vi "Process.vi"(8 "error in":errorcluster, 11 "LockinDAQ":refnum<class "Lockin.DAQ.lvclass">) -> (0 "error out":errorcluster, 3 "LockinDAQ out":refnum<class "Lockin.DAQ.lvclass">)   [LabVIEW 2016, in "Lockin.DAQ.lvclass"]
doc: "---------------------------------------------------------------\nJKI State Machine Objects™\nhttp://jki.net/state-machine-objects/\nCopyright (C) 2005-2015, JKI <info@jki.net>\nALL RIGHTS RESERVED"
uses:
  Lockin.DAQ.lvclass
  C:/Program Files (x86)/National Instruments/LabVIEW 2016/vi.lib/JKI/JKI SMO/SMO/SMO.lvclass
  Typedefs/State-enum.ctl
  <vilib>/JKI/JKI SMO/SMO/Typedefs/Parent Call--Enum.ctl
  Lockin.DAQ.lvclass/Lockin.DAQ.ctl
  Typedefs/Results--Cluster.ctl
  Typedefs/Sample Mode--Ring.ctl
  Typedefs/SweepResults--Cluster.ctl
  Typedefs/PublicEvents--Lockin.DAQ.getSweepWaveforms.ctl
  Typedefs/PrivateEvents--Cluster.ctl
  Typedefs/PrivateEvents--Lockin.DAQ.setAOconfig.ctl
  Typedefs/AO.config-array.ctl
  Typedefs/AO.config-cluster.ctl
  Typedefs/446xAO-enum.ctl
  Typedefs/DAQType-enum.ctl
  Typedefs/PrivateEvents--Lockin.DAQ.setAIconfig.ctl
  Typedefs/AI.config-array.ctl
  Typedefs/AI.config-cluster.ctl
  Typedefs/AI.coupling-enum.ctl
  Typedefs/446xAI-enum.ctl
  Typedefs/AI Simulation-enum.ctl
  Typedefs/PrivateEvents--Lockin.DAQ.setAO.ctl
  Typedefs/AO-cluster.ctl
  Instrument.Lockinl.UI/Typedefs/AO Channel--Cluster.ctl
  Typedefs/Function-enum.ctl
  Typedefs/PrivateEvents--Lockin.DAQ.setREF.ctl
  Typedefs/REF-cluster.ctl
  Instrument.Lockinl.UI/Typedefs/REF Channel--Cluster.ctl
  Typedefs/PrivateEvents--Lockin.DAQ.setSampling.ctl
  Typedefs/Sampling.ctl
  Typedefs/PrivateEvents--Lockin.DAQ.setState.ctl
  Typedefs/Set State-enum.ctl
  Typedefs/PrivateEvents--Lockin.DAQ.setInputGain.ctl
  Typedefs/PrivateEvents--Lockin.DAQ.setSweep.ctl
  Typedefs/Sweep Configuration--Cluster.ctl
  Instrument.Lockinl.UI/Typedefs/Sweep Channel--Cluster.ctl
  Typedefs/Sweep Pattern--Enum.ctl
  Typedefs/PrivateEvents--Lockin.DAQ.measureOffset.ctl
  Typedefs/PrivateEvents--Lockin.DAQ.zeroOffset.ctl
  Typedefs/PrivateEvents--Lockin.DAQ.setPreFilter.ctl
  Typedefs/AI Prefilter-cluster.ctl
  Typedefs/PrivateEvents--Lockin.DAQ.autoContigureDAQ.ctl
  Typedefs/PrivateEvents--LockinDAQ.setCalibration.ctl
  Typedefs/PrivateEvents--Lockin.DAQ.setAI.ctl
  Typedefs/AI-cluster.ctl
  Instrument.Lockinl.UI/Typedefs/AI Channel--Cluster.ctl
  Typedefs/PrivateEvents--Lockin.DAQ.Reset Phase.ctl
  <vilib>/JKI/JKI SMO/SMO/Typedefs/Protected Events.ctl
  <vilib>/JKI/JKI SMO/SMO/Typedefs/StopProcessEventData--Cluster.ctl
  <vilib>/JKI/JKI SMO/SMO/Typedefs/AbortProcessEventData--Cluster.ctl
  <vilib>/JKI/JKI SMO/SMO/Typedefs/SMO Dependency Event--Cluster.ctl
  <vilib>/JKI/JKI SMO/SMO/Typedefs/SMO Dependency Event--Enum.ctl
  <vilib>/Analysis/2dsp.llb/Decimate (single shot).vi
  <vilib>/Analysis/2dsp.llb/Decimate (single shot, DBL).vi
  <vilib>/Utility/High Resolution Relative Seconds.vi
  <vilib>/Waveform/WDTOps.llb/Number of Waveform Samples.vi
  <vilib>/Waveform/WDTOps.llb/WDT Number of Waveform Samples DBL.vi
  <vilib>/measure/madcrms.llb/Basic Averaged DC-RMS for N Chan.vi
  <vilib>/JKI/JKI SMO/SMO/SMO.lvclass
  <resource>/objmgr/daqmx.rc
  Instrument.Lockin/Instrument.Lockin.lvclass
  <vilib>/measure/NI_MAPro.lvlib
  Instrument.Lockinl.UI/Instrument.Lockin.UI.lvclass
panel:
  in  "Tab Control":enum32{"SMO", "Other", "Sweeping"}(tab)
  out "DAQ state":T1=enum."created"
  out "Method":string
  out "to":i32
  in  "LP Cutoff (Hz)":dbl=0.45 format="%#_13g"
  in  "LP filter?":bool
  in  "60 Hz Prefilter?":bool
  in  "reset REF":bool
  out "DAQ Create Tasks (ms)":u32
  out "DAQ AO/AI (ms)":u32
  out "Lockin (ms)":u32
  out "WFM Generation (ms)":u32
  out "DAQ Start Tasks (ms)":u32
  out "Payload":variant
  out "State":string
  in  "measure offset":bool
  in  "zero offset":bool
  in  "Reset Phase?":bool
  in  "autophase?\n(experimental)":bool
  out "ms":u32
  out "Sweeping Time":timestamp
  out "Sweep Start":timestamp
  out "Sweep Wait Time":timestamp
  out "sweeping":dbl
  out "sweep index":i32
  out "waiting (s)":dbl
  out "done sweep?":bool
  out "timeout?":bool
  # "For instructions on how to use the JKI State Machine Objects, examples and video tutorials, visit:\nhttp://jki.net/state-machine-objects/\n\nJKI State Machine Objects™\nhttp://jki.net/state-machine-objects/\nCopyright (C) 2005-2015, JKI <info@jki.net>\nALL RIGHTS RESERVED"
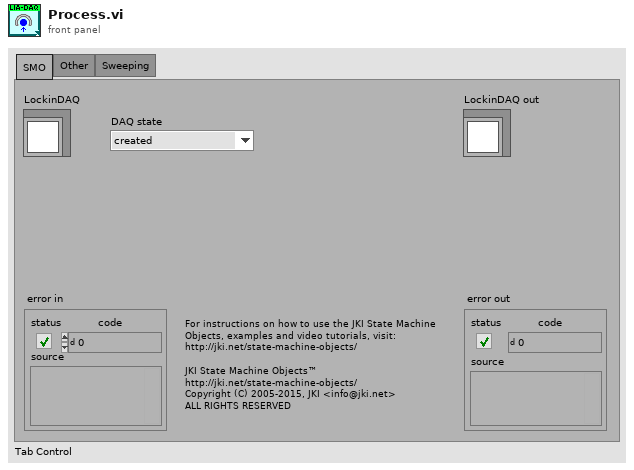
[diagram p1: front panel]
types:
  T1 = typedef "Lockin.DAQ.lvclass/State-enum.ctl" = enum16{"idle", "created", "started", "stopped", "sweeping"}
  T2 = typedef "SMO.lvclass/Parent Call--Enum.ctl" = enum16{"Allows parent to run", "Does not request parent to run"}
  T3 = enum32{"invalid app kind", "Development System", "Run Time System", "Student Edition", "Embedded LabVIEW", "Evaluation", "Custom"}
  T4 = enum32{"Invalid", "Standard", "Closed", "Hidden", "Minimized", "Maximized"}
  T5 = enum32{"Bad", "Idle", "Run top level", "Running"}
  T6 = typedef "Lockin.DAQ.lvclass/SweepResults--Cluster.ctl" = cluster{"X results":waveform(dbl)[], "Y Results":waveform(dbl)[]}
  T7 = typedef "Lockin.DAQ.lvclass/Sample Mode--Ring.ctl" = i32
  T8 = typedef "Lockin.DAQ.lvclass/AO.config-array.ctl" = T9[]
  T9 = typedef "Lockin.DAQ.lvclass/AO.config-cluster.ctl" = cluster{"AO.channels":tag, "AO.Range":T10, "output terminal configuration":i32, "DAQ Type":T11}
  T10 = typedef "Lockin.DAQ.lvclass/446xAO-enum.ctl" = enum16{"±0.1", "±1.0", "±10.0"}
  T11 = typedef "Lockin.DAQ.lvclass/DAQType-enum.ctl" = enum16{"None", "USB 4431", "PXI 446x"}
  T12 = typedef "Lockin.DAQ.lvclass/Results--Cluster.ctl" = cluster{"Time Stamp":timestamp, "Results":dbl[][]}
  T13 = cluster{"Core":cluster{"Current VI Reference":refnum<vi>, "Close Panel on Exit?":bool, "error":errorcluster}, "Self Reference":refnum<class "Lockin.DAQ.lvclass">, "to":i32, "state":T1, "sample mode":T7, "AO":waveform(dbl)[], "AI":waveform(dbl)[], "Reference":cluster{"X":waveform(dbl)[], "Y":waveform(dbl)[]}, "Results":T12, "sweep index":i32, "SweepResults [i]":T6, "SweepResults []":T6, "DAQ Offset":dbl[], "Sweep_AO":waveform(dbl)[], "Sweep_AI":waveform(dbl)[], "Reset Phase":bool, "Measure Offset":bool}
  T14 = typedef "Lockin.DAQ.lvclass/AI.config-array.ctl" = T15[]
  T15 = typedef "Lockin.DAQ.lvclass/AI.config-cluster.ctl" = cluster{"AI.channels":tag, "AI.Coupling":T16, "AI.Range":T17, "input terminal configuration":i32, "DAQ Type":T11}
  T16 = typedef "Lockin.DAQ.lvclass/AI.coupling-enum.ctl" = u16
  T17 = typedef "Lockin.DAQ.lvclass/446xAI-enum.ctl" = enum16{"±0.316", "±1.00", "±3.16", "±10.0", "±31.6", "±42.4"}
  T18 = typedef "Lockin.DAQ.lvclass/AI Simulation-enum.ctl" = enum16{"AI = HW simulated", "AI = noise*AO", "AI = waveguide"}
  T19 = cluster{"AI Configuration":T14, "Simulation mode":T18}
  T20 = typedef "Lockin.DAQ.lvclass/AO-cluster.ctl" = T21[]
  T21 = typedef "Instrument.Lockin.UI.lvclass/AO Channel--Cluster.ctl" = cluster{"Enable?":bool, "Channel":i32, "Amplitude":dbl, "Offset":dbl, "Frequency":dbl, "Phase":dbl, "Function":T22, "Sweeping?":bool}
  T22 = typedef "Lockin.DAQ.lvclass/Function-enum.ctl" = enum16{"Sine", "Triangle", "Square"}
  T23 = typedef "Lockin.DAQ.lvclass/AI-cluster.ctl" = T24[]
  T24 = typedef "Instrument.Lockin.UI.lvclass/AI Channel--Cluster.ctl" = cluster{"Enable?":bool, "Channel":i32, "References":u16[]}
  T25 = typedef "Lockin.DAQ.lvclass/REF-cluster.ctl" = T26[]
  T26 = typedef "Instrument.Lockin.UI.lvclass/REF Channel--Cluster.ctl" = cluster{"Enable?":bool, "Channel":i32, "Frequency":dbl, "Phase":dbl, "TC":dbl, "Order":i32}
  T27 = typedef "Lockin.DAQ.lvclass/PrivateEvents--Lockin.DAQ.setInputGain.ctl" = dbl[]
  T28 = typedef "Lockin.DAQ.lvclass/Sampling.ctl" = cluster{"Fs":dbl, "#s":i32}
  T29 = cluster{"Sampling":T28, "Sample Mode":T7, "AI Buffer Size (S)":i32, "Decimation":i32}
  T30 = typedef "Lockin.DAQ.lvclass/Sweep Configuration--Cluster.ctl" = cluster{"Sweep Time (s)":dbl, "Initial Wait (s)":dbl, "Return to Start":bool, "Channels":T31[]}
  T31 = typedef "Instrument.Lockin.UI.lvclass/Sweep Channel--Cluster.ctl" = cluster{"End":dbl, "Start":dbl, "Channel":u16, "Pattern":T32}
  T32 = typedef "Lockin.DAQ.lvclass/Sweep Pattern--Enum.ctl" = enum16{"Ramp /", "Ramp /\\", "Smooth Ramp _/", "Smooth Ramp _/\\_", "Frequency"}
  T33 = typedef "Lockin.DAQ.lvclass/PrivateEvents--Lockin.DAQ.measureOffset.ctl" = bool
  T34 = typedef "Lockin.DAQ.lvclass/PrivateEvents--Lockin.DAQ.Reset Phase.ctl" = bool
  T35 = typedef "Lockin.DAQ.lvclass/AI Prefilter-cluster.ctl" = cluster{"60 Hz prefilter":bool, "LP prefilter":bool, "LP cutoff (Hz)":dbl}
  T36 = typedef "Lockin.DAQ.lvclass/Set State-enum.ctl" = enum16{"start", "stop", "reset", "start sweep", "stop sweep"}
  T37 = typedef "Lockin.DAQ.lvclass/PrivateEvents--LockinDAQ.setCalibration.ctl" = bool
  T38 = cluster{"X":waveform(dbl)[], "Y":waveform(dbl)[]}
  T39 = typedef "Lockin.DAQ.lvclass/PublicEvents--Lockin.DAQ.getSweepWaveforms.ctl" = cluster{"Sweep_AO":waveform(dbl)[], "Sweep_AI":waveform(dbl)[]}
  T40 = cluster{"Current VI Reference":refnum<vi>, "Close Panel on Exit?":bool, "error":errorcluster}
  T41 = typedef "SMO.lvclass/Protected Events.ctl" = cluster{"StopProcesses":refnum<user-event>, "AbortProcesses":refnum<user-event>, "Config Changed":refnum<user-event>, "Dependency":refnum<user-event>}
  T42 = typedef "Lockin.DAQ.lvclass/PrivateEvents--Cluster.ctl" = cluster{"setAOconfig":refnum<user-event>, "setAIconfig":refnum<user-event>, "setAO":refnum<user-event>, "setREF":refnum<user-event>, "setSampling":refnum<user-event>, "setState":refnum<user-event>, "setInputGain":refnum<user-event>, "setOutputGain":refnum<user-event>, "setSweep":refnum<user-event>, "measureOffset":refnum<user-event>, "zeroOffset":refnum<user-event>, "setPreFilter":refnum<user-event>, "autoConfigureDAQ":refnum<user-event>, "setCalibration":refnum<user-event>, "setAI":refnum<user-event>, "Reset Phase":refnum<user-event>}
  T43 = cluster{"SMO":refnum<event-registration>, "LockinDAQ":refnum<event-registration>, "DAQmx":refnum<event-registration>}
  T44 = typedef "Instrument.Lockin.UI.lvclass/Device Configuration--Cluster.ctl" = cluster{"Device":string, "AO.Ch":string, "AO.Range":T10, "AI.Ch":string, "AI.Range":T17, "AI.Coupling":T16}
  T45 = typedef "Lockin.DAQ.lvclass/Cal Info - Cluster.ctl" = cluster{"Active Device":string, "SelfCal.LastDate/Time":dbl, "SelfCal.LastTemp":dbl, "DevTemp":dbl, "calibration due?":bool}
  T46 = cluster{"Array out":waveform(dbl)[], "Array out":waveform(dbl)[]}
  T47 = cluster{"Sweep_AO":waveform(dbl)[], "Sweep_AI":waveform(dbl)[]}
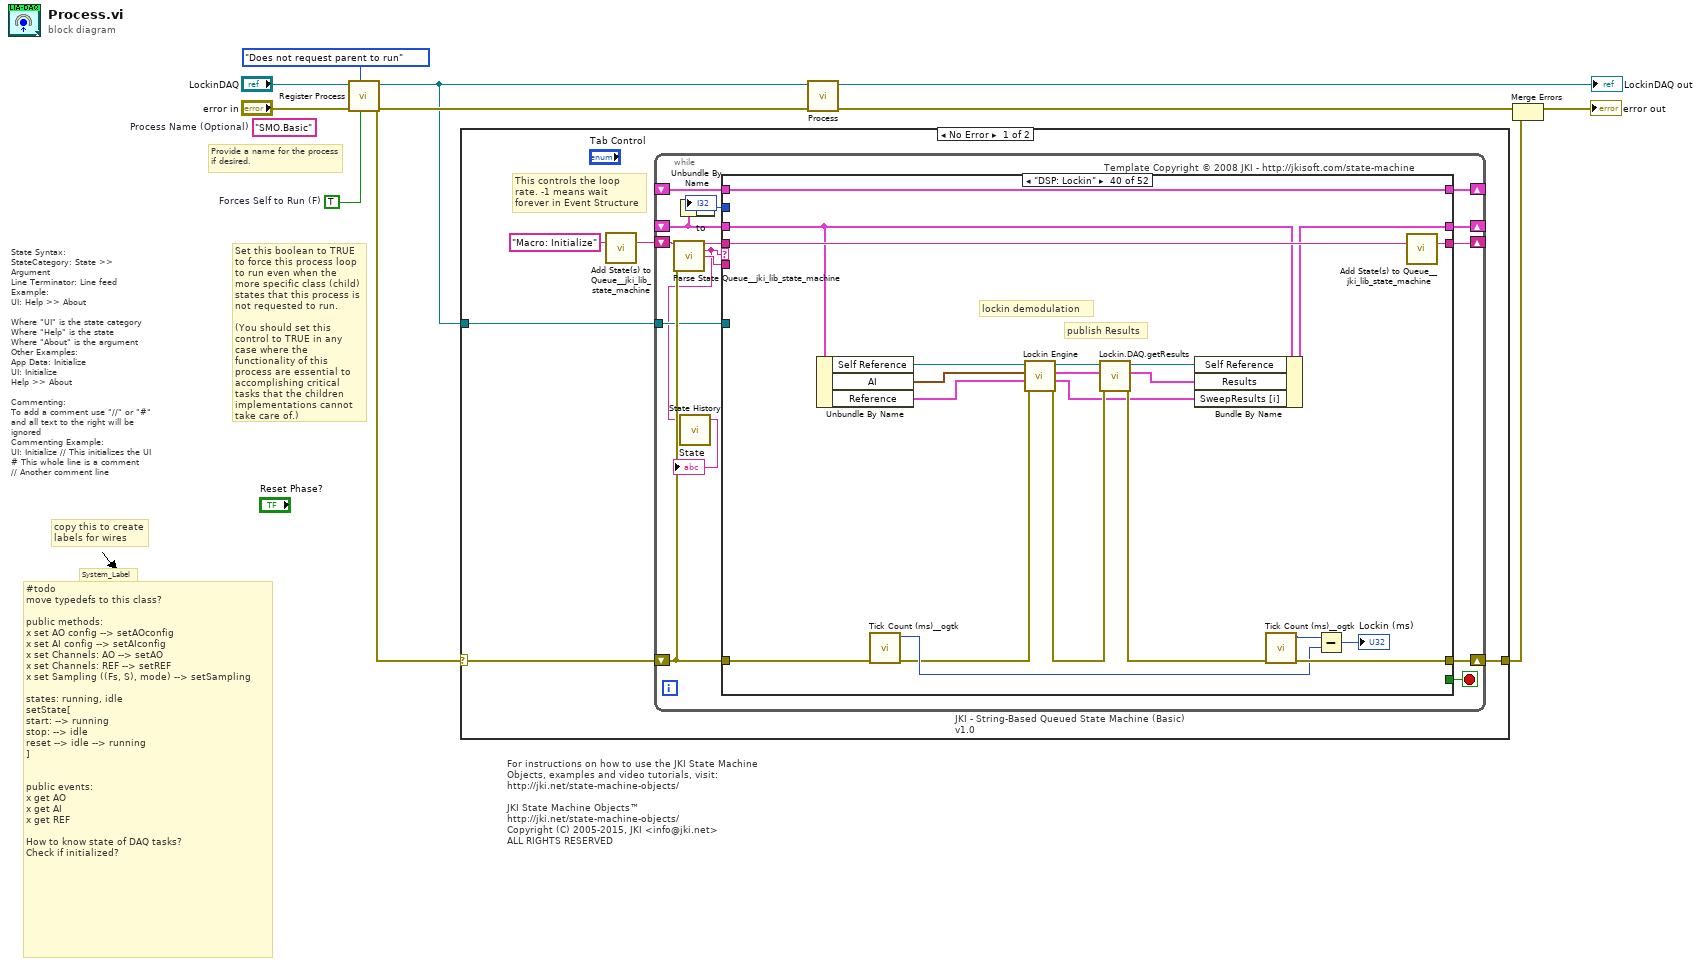
[diagram p0: block diagram]
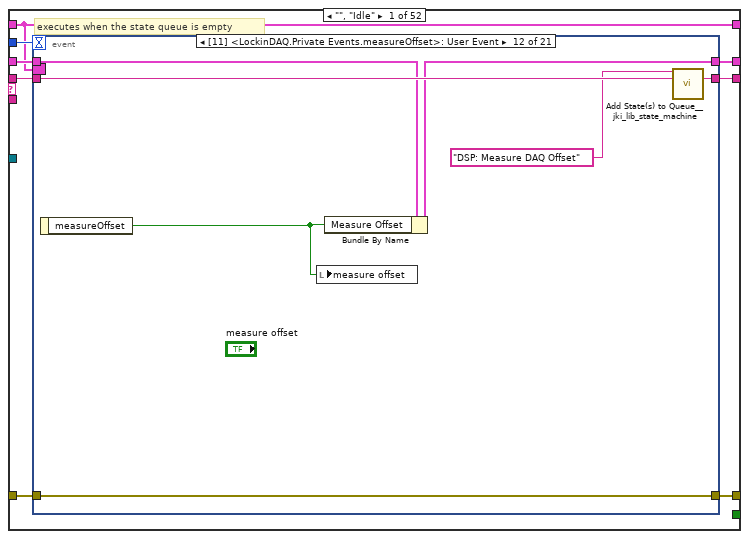
[diagram p2: hidden frame]
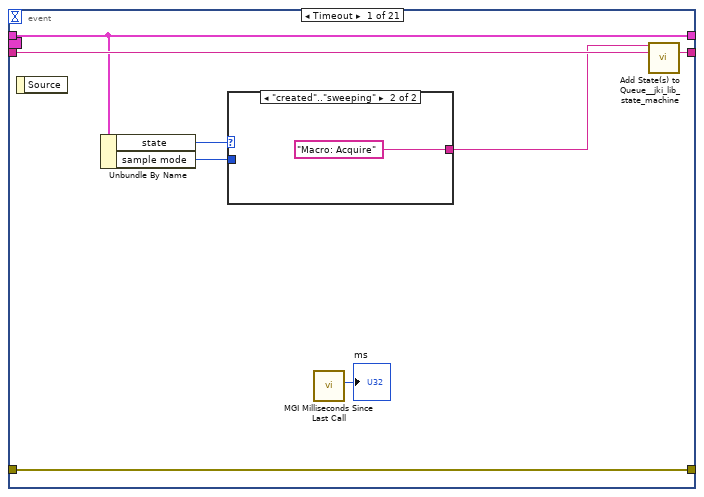
[diagram p3: hidden frame]
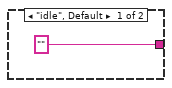
[diagram p4: hidden frame]
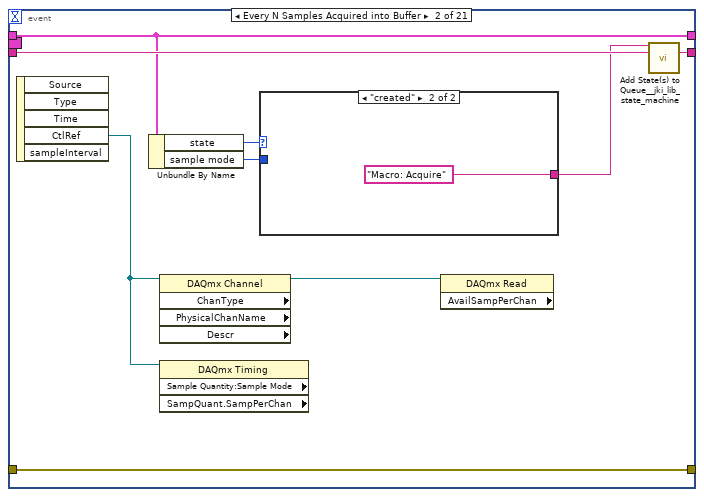
[diagram p5: hidden frame]
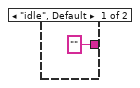
[diagram p6: hidden frame]
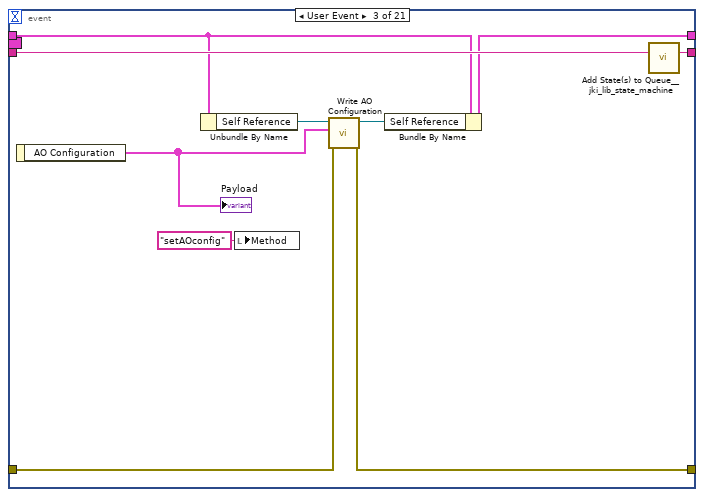
[diagram p7: hidden frame]
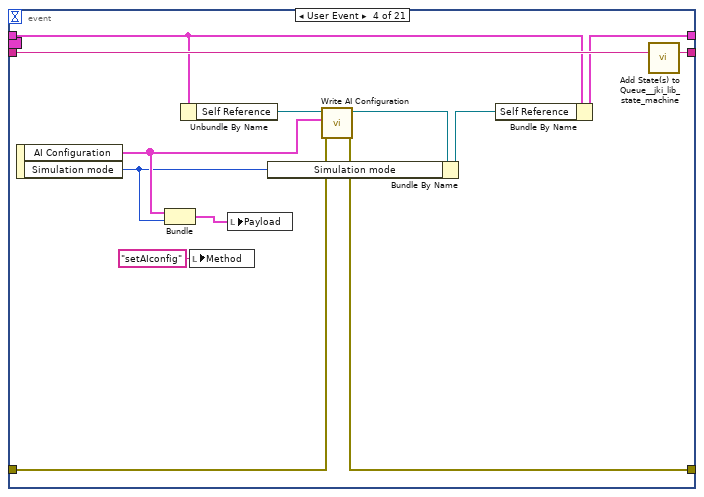
[diagram p8: hidden frame]
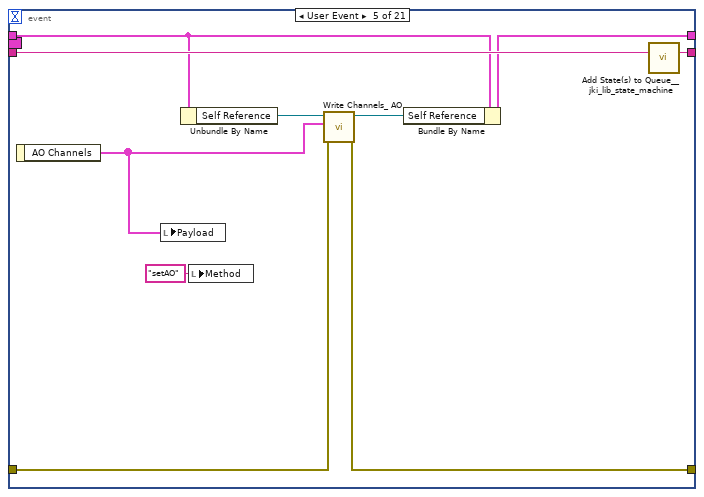
[diagram p9: hidden frame]
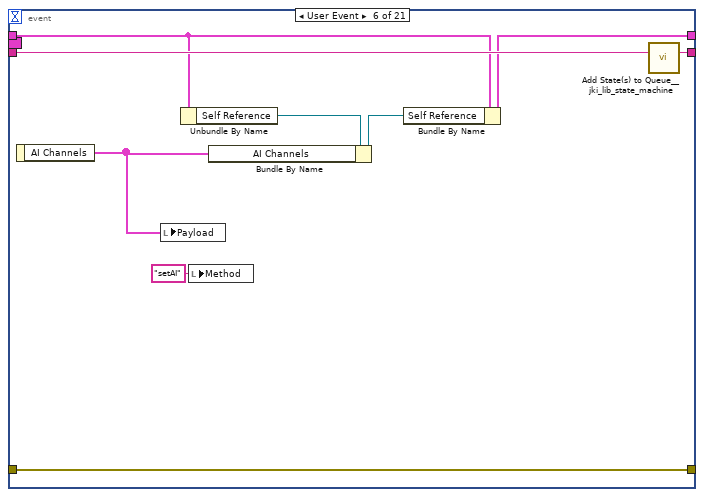
[diagram p10: hidden frame]
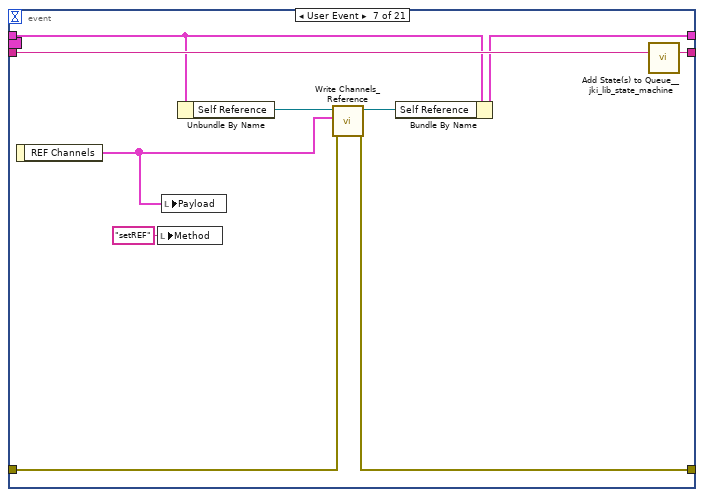
[diagram p11: hidden frame]
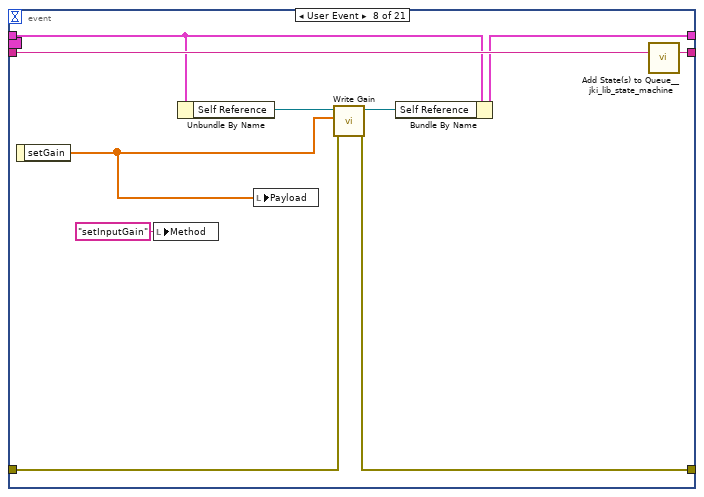
[diagram p12: hidden frame]
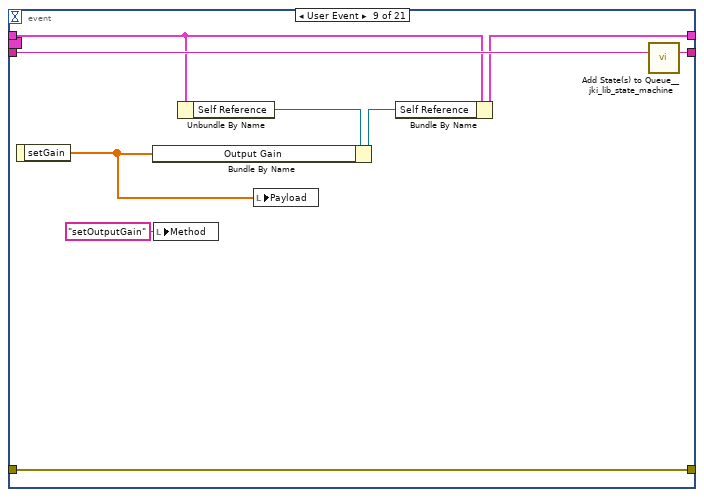
[diagram p13: hidden frame]
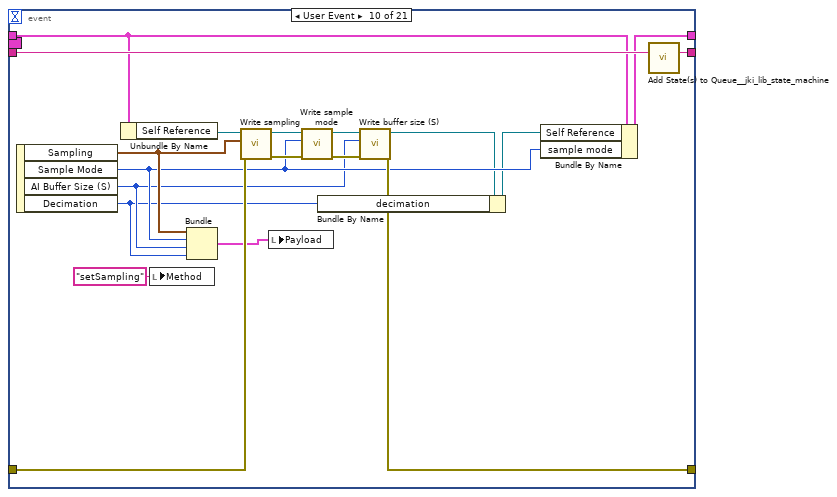
[diagram p14: hidden frame]
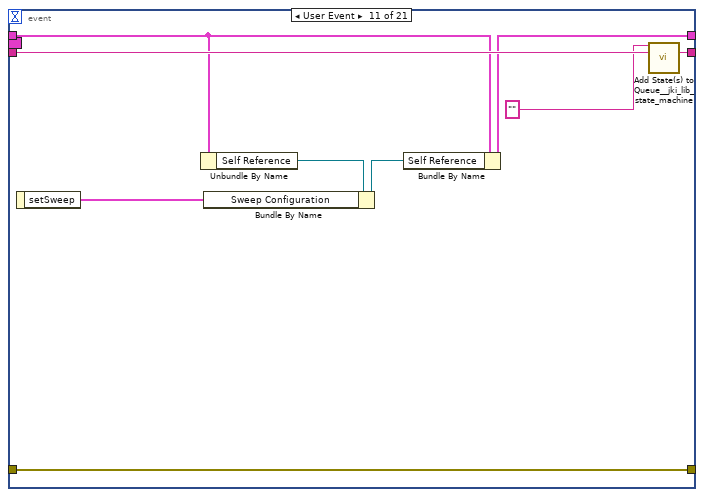
[diagram p15: hidden frame]
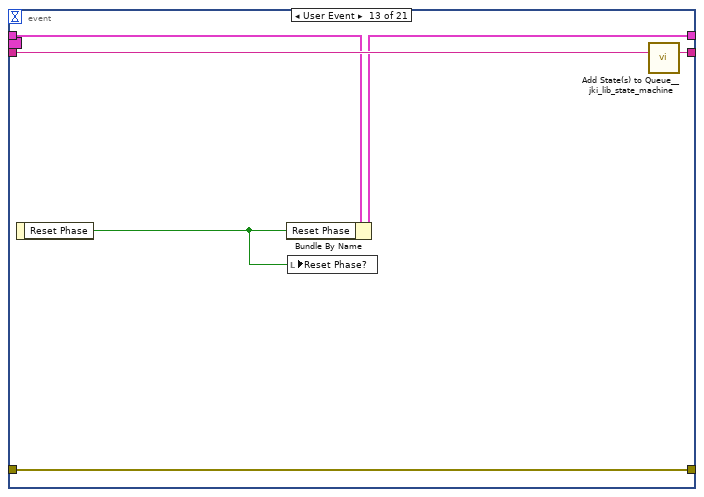
[diagram p16: hidden frame]
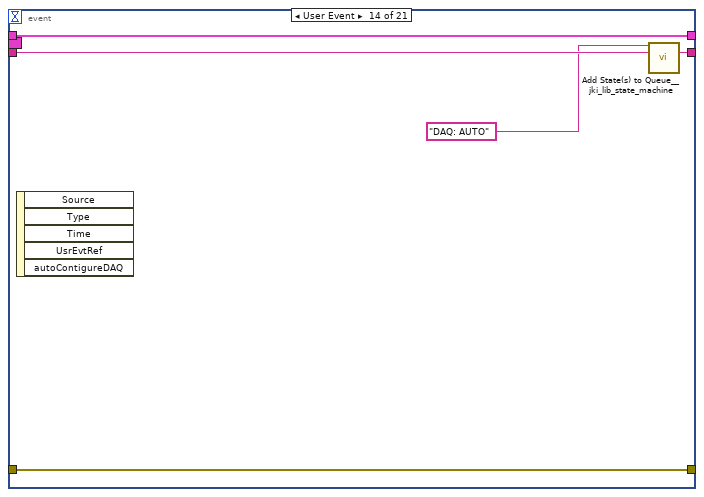
[diagram p17: hidden frame]
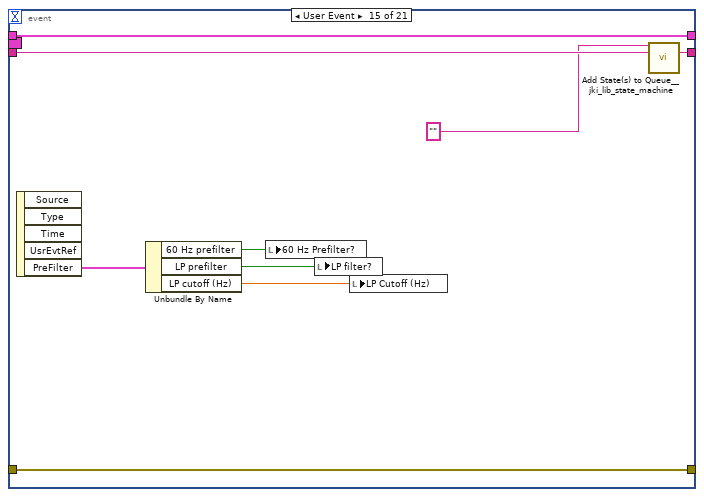
[diagram p18: hidden frame]
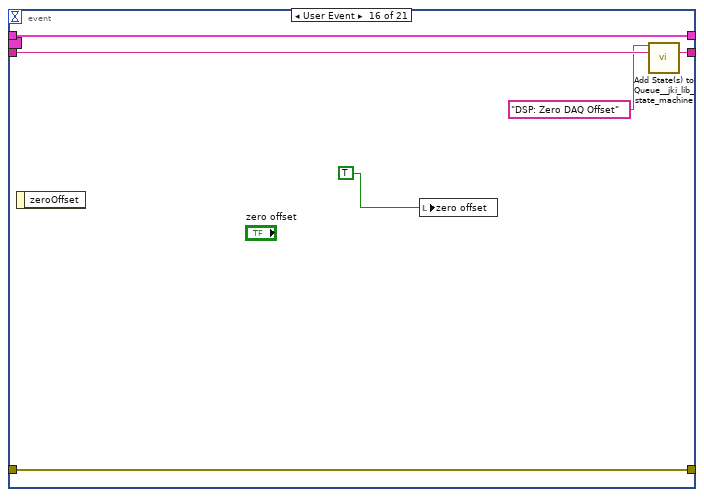
[diagram p19: hidden frame]
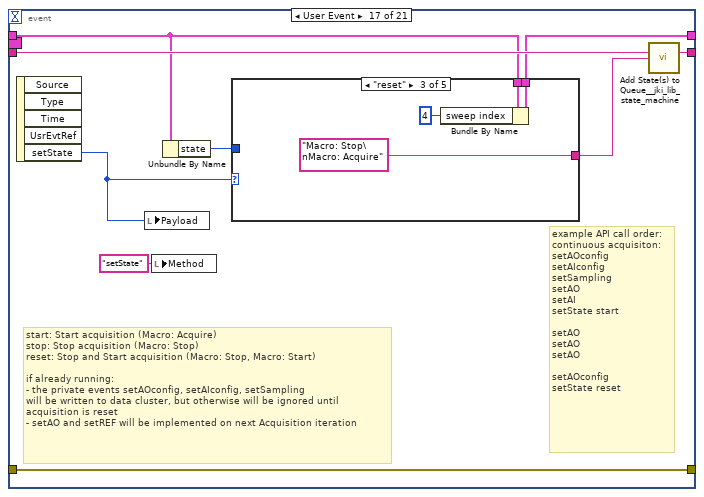
[diagram p20: hidden frame]
diagram:
  w1 = TRUE  # Forces Self to Run (F)
  (unwired) "SMO.Basic"  # Process Name (Optional)
  # "State Syntax:\nStateCategory: State >> Argument\nLine Terminator: Line feed\nExample:\nUI: Help >> About\n\nWhere \"UI\" is the state category\nWhere \"Help\" is the state\nWhere \"About\" is the argument\nOther Examples:\nApp Data: Initialize\nUI: Initialize\nHelp >> About\n\nCommenting:\nTo add a comment use \"//\" or \"#\" and all text to the right will be ignored\nCommenting Example:\nUI: Initialize // This initializes the UI\n# This whole line is a comment\n// Another comment line"
  # "copy this to create labels for wires"
  # "System_Label"
  # "#todo\nmove typedefs to this class?\n\npublic methods:\nx set AO config --> setAOconfig\nx set AI config --> setAIconfig\nx set Channels: AO --> setAO\nx set Channels: REF --> setREF\nx set Sampling ((Fs, S), mode) --> setSampling\n\nstates: running, idle\nsetState[\nstart: --> running\nstop: --> idle\nreset --> idle --> running\n]\n\n\npublic events:\nx get AO\nx get AI\nx get REF\n\nHow to know state of DAQ tasks?\nCheck if initialized?"
  # "Provide a name for the process\nif desired."
  # "Set this boolean to TRUE to force this process loop to run even when the more specific class (child) states that this process is not requested to run.\n\n(You should set this control to TRUE in any case where the functionality of this process are essential to accomplishing critical tasks that the children implementations cannot take care of.)"
  # "For instructions on how to use the JKI State Machine Objects, examples and video tutorials, visit:\nhttp://jki.net/state-machine-objects/\n\nJKI State Machine Objects™\nhttp://jki.net/state-machine-objects/\nCopyright (C) 2005-2015, JKI <info@jki.net>\nALL RIGHTS RESERVED"
  n1 = call <vilib>:"Register Process.vi"("Forces Self to Run (F)"=w1, "Parent Call"=Parent_Call--Enum."Does not request parent to run", "error in (no error)"="error in", "SMO"="LockinDAQ") -> ("error out"=w7:errorcluster, "SMO out"=w6:refnum<class "Lockin.DAQ.lvclass">)  [unwired: 6 in]
  n2 = case shown="No Error" w7 {
    selector: w7 -> [w14 w1097]
    tunnel: w6 -> [w15 _]
    tunnel: [w13 w1097] -> w3
    frame No Error {
      # "This controls the loop rate. -1 means wait forever in Event Structure"
      n3 = call <vilib>:"Add State(s) to Queue__jki_lib_state_machine.vi"("State(s) in (\"\")"="Macro: Initialize") -> ("States Out"=w12:string)  [unwired: 14 in]
      n4 = while "JKI - String-Based Queued State Machine (Basic) v1.0" {
        shift-right: [w25] -> _
        shift-left: _ -> [w19]
        shift-right: [w18] -> w13
        shift-left: w14 -> [w24]
        shift-right: [w27] -> _
        shift-left: w12 -> [w28]
        tunnel: w15 -> [w23]
        shift-right: [w22] -> _
        shift-left: _ -> [w21]
        stop <- w26 stop-if-true
        # "Template Copyright © 2008 JKI - http://jkisoft.com/state-machine"
        n5 = call <vilib>:"Parse State Queue__jki_lib_state_machine.vi"("State Queue"=w28, "Error In (no error)"=w24) -> ("Remaining States"=w30:string, "Current State"=w16:string, "Arguments"=w29:string)  [unwired: 11 in]
        n6 = call "State History.vi"("Current State in"=w16) -> ("State History"=→"State":string)  [unwired: 4 in]
        n7 = Unbundle By Name(w19) -> ("to"=w20:i32)
        "to" <- w20
        n8 = case shown="\"DSP: Lockin\"" w16 {
          selector: w16 -> [_ _ w253 _ _ _ _ _ _ _ _ _ _ _ _ _ _ _ _ _ _ _ _ _ _ _ _ _ _ _ _ _ _ _ _ _ _ _ _ _ _ _ _ _ _ _ _ _ _ _ _ _]
          tunnel: w30 -> [w38 w251 w257 w276 _ w303 w308 w334 w341 w346 w352 w359 w375 w407 w421 w436 w449 w459 w467 w475 w487 w492 w503 w508 w531 w537 w542 w559 w593 w611 w650 w659 w672 w695 w732 w744 w749 w765 w827 w899 w915 w924 w930 w943 w950 w969 w978 w1000 w1028 w1069 w1074 w1082]
          tunnel: w29 -> [_ _ _ _ _ _ _ _ _ _ _ w353 w369 _ _ _ _ _ _ _ _ _ _ _ _ _ _ _ _ _ _ _ w667 _ _ _ _ _ _ _ _ _ _ _ _ _ _ _ _ _ _ _]
          tunnel: w19 -> [w36 w248 w255 w267 w295 w299 w305 _ w335 w343 w350 w357 w371 w404 w417 w428 w444 w456 w460 w472 w485 w489 w500 w505 w529 w535 w540 w556 w588 w608 w647 w657 w669 w692 w729 w737 w747 w755 w824 w896 w912 w918 w928 w940 w944 w960 w975 w997 w1022 w1065 w1072 w1094]
          tunnel: w24 -> [w34 w249 w258 w273 w278 _ w306 w332 w338 w344 w349 w355 w373 w405 w419 w434 w447 w457 w465 w468 w486 w490 w495 w506 w527 w534 w538 w553 w589 w605 w645 w652 w665 w689 w726 w739 w745 w750 w802 w894 w905 w921 w926 w935 w945 w958 w972 w990 w1014 w1063 w1070 w1091]
          tunnel: [w37 w250 w256 w275 w285 w302 w307 w333 w340 w345 w351 w358 w374 w406 w420 w435 w448 w458 w466 w474 w483 w491 w502 w507 w530 w536 w541 w558 w592 w610 w649 w658 w671 w694 w731 w743 w748 w764 w826 w898 w914 w923 w929 w942 w949 w968 w977 w999 w1027 w1068 w1073 w1096] -> w27
          tunnel: [_ _ _ _ _ TRUE _ _ _ _ _ _ _ _ _ _ _ _ _ _ _ _ _ _ _ _ _ _ _ _ _ _ _ _ _ _ _ _ _ _ _ _ _ _ _ _ _ _ _ _ _ _] -> w26
          tunnel: [w33 w248 w255 w274 w294 w299 w305 w324 w335 w343 w350 w357 w371 w404 w417 w428 w444 w456 w460 w472 w485 w489 w500 w505 w529 w535 w540 w555 w587 w607 w646 w656 w668 w691 w728 w736 w747 w754 w823 w895 w911 w920 w928 w939 w944 w959 w974 w996 w1021 w1066 w1072 w1093] -> w25
          tunnel: w20 -> [w32 _ _ _ _ _ _ _ _ _ _ _ _ _ _ _ _ _ _ _ _ _ _ _ _ _ _ _ _ _ _ _ _ _ _ _ _ _ _ _ _ _ _ _ _ _ _ _ _ _ _ _]
          tunnel: w23 -> [_ _ _ _ _ _ _ w330 _ _ _ _ _ _ _ _ _ _ _ _ _ _ _ _ _ _ _ _ _ _ _ _ _ _ _ _ _ _ _ _ _ _ _ _ _ _ _ _ _ _ _ _]
          tunnel: [w31 w247 w252 w264 w297 w300 w304 w329 w336 w342 w348 w356 w368 w403 w418 w429 w446 w455 w464 w473 w484 w488 w501 w504 w522 w532 w539 w557 w591 w609 w648 w655 w670 w693 w730 w741 w746 w763 w825 w897 w913 w922 w927 w941 w948 w967 w976 w998 w1026 w1067 w1071 w1095] -> w22
          tunnel: w21 -> [w31 w247 w252 w264 w297 w300 w304 w329 w336 w342 w348 w356 w368 w403 w418 w429 w446 w455 w464 w473 w484 w488 w501 w504 _ w532 w539 w557 w591 w609 w648 w655 w670 w693 w730 w740 w746 w763 w825 w897 w913 w922 w927 w941 w948 w967 w976 w998 w1026 w1067 w1071 w1095]
          tunnel: [w35 w249 w259 w273 w296 w298 w306 w319 w337 w344 w349 w354 w372 w405 w419 w434 w447 w457 w465 w468 w486 w490 w494 w506 w526 w534 w538 w552 w582 w604 w639 w651 w660 w684 w720 w738 w745 w753 w818 w889 w909 w921 w926 w938 w946 w958 w972 w991 w1015 w1064 w1070 w1088] -> w18
          frame "", "Idle" {
            # "executes when the state queue is empty"
            n9 = event shown="[11] <LockinDAQ.Private Events.measureOffset>: User Event" {
              selector: w31 -> [_ _ _ _ _ _ _ _ _ _ _ _ _ _ _ _ _ _ _ _ _]
              dyn-events: _ -> [_ _ _ _ _ _ _ _ _ _ _ _ _ _ _ _ _ _ _ _ _]
              timeout: w32 -> [_ _ _ _ _ _ _ _ _ _ _ _ _ _ _ _ _ _ _ _ _]
              tunnel: w38 -> [w46 w57 w69 w82 w92 w101 w111 w121 w130 w149 w158 w165 w171 w176 w185 w191 w200 w230 w236 w241 w246]
              tunnel: [w45 w56 w68 w81 w91 w100 w110 w120 w129 w148 w157 w164 w170 w175 w184 w190 w199 w229 w235 w240 w245] -> w37
              tunnel: w36 -> [w43 w54 w65 w78 w88 w97 w107 w117 w126 w145 w154 w161 w168 w172 w181 w188 w193 w225 w233 w238 w243]
              tunnel: [w44 w55 w61 w75 w84 w93 w103 w114 w125 w138 w155 w163 w169 w174 w183 w189 w198 w228 w234 w239 w244] -> w35
              tunnel: w34 -> [w44 w55 w62 w76 w85 w93 w104 w115 w125 w141 w155 w163 w169 w174 w183 w189 w198 w228 w234 w239 w244]
              tunnel: [w43 w54 w67 w80 w90 w99 w109 w119 w128 w147 w156 w160 w167 w172 w181 w188 w192 w225 w233 w238 w243] -> w33
              event Timeout {
                n10 = event-data() -> ()  [unwired: 1 in, 1 out]
                n11 = Unbundle By Name(w43) -> ("state"=w41:T1, "sample mode"=w42:T7)
                n12 = case shown="\"created\"..\"sweeping\"" w41 {
                  tunnel: w42 -> [_ _]
                  tunnel: ["" ("State(s) in Front (\"\")") "Macro: Acquire" ("State(s) in Front (\"\")")] -> w40
                  frame "idle", Default {
                  }
                  frame "created".."sweeping" {
                  }
                }
                n13 = call <userlib>:"MGI Milliseconds Since Last Call.vi"() -> ("ms"=→"ms":u32)  [unwired: 6 in, 1 out]
                n14 = call <vilib>:"Add State(s) to Queue__jki_lib_state_machine.vi"("State(s) in Front (\"\")"=w40, "State(s) in (\"\")"=w46) -> ("States Out"=w45:string)  [unwired: 13 in]
              }
              event Every N Samples Acquired into Buffer {
                n15 = event-data() -> ("CtlRef"=w50:refnum<k21>)  [unwired: 1 in, 4 out]
                n16 = Unbundle By Name(w54) -> ("state"=w51:T1, "sample mode"=w53:T7)
                n17 = property class="DAQmx Channel" props=["ChanType", "PhysicalChanName", "Descr"](reference=w50) -> (reference out=w49:refnum<k21>)  [unwired: 1 in, 4 out]
                n18 = property class="DAQmx Timing" props=["Sample Quantity:Sample Mode", "SampQuant.SampPerChan"](reference=w50) -> ()  [unwired: 1 in, 4 out]
                n19 = case shown="\"created\"" w51 {
                  tunnel: w53 -> [_ _]
                  tunnel: ["" ("State(s) in Front (\"\")") "Macro: Acquire" ("State(s) in Front (\"\")")] -> w52
                  frame "idle", Default {
                  }
                  frame "created" {
                  }
                }
                n20 = property class="DAQmx Read" props=["AvailSampPerChan"](reference=w49) -> ()  [unwired: 1 in, 3 out]
                n21 = call <vilib>:"Add State(s) to Queue__jki_lib_state_machine.vi"("State(s) in Front (\"\")"=w52, "State(s) in (\"\")"=w57) -> ("States Out"=w56:string)  [unwired: 13 in]
              }
              event User Event {
                n22 = event-data() -> ("AO Configuration"=w60:T8)  [unwired: 1 in]
                "Payload" <- w60
                n23 = Unbundle By Name(w65) -> ("Self Reference"=w64:refnum<class "Lockin.DAQ.lvclass">)
                n24 = local write "Method"("setAOconfig" ("String")) -> ()
                n25 = call "Write AO Configuration.vi"("error in (no error)"=w62, "AO Configuration"=w60, "Lockin.DAQ"=w64) -> ("error out"=w61:errorcluster, "Lockin.DAQ out"=w63:refnum<class "Lockin.DAQ.lvclass">)  [unwired: 7 in]
                n26 = Bundle By Name(cluster=w65, "Self Reference"=w63) -> (w67:T13)
                n27 = call <vilib>:"Add State(s) to Queue__jki_lib_state_machine.vi"("State(s) in (\"\")"=w69) -> ("States Out"=w68:string)  [unwired: 14 in]
              }
              event User Event {
                n28 = event-data() -> ("AI Configuration"=w72:T14, "Simulation mode"=w71:T18)  [unwired: 1 in]
                n29 = Bundle("AI Configuration"=w72, "Simulation mode"=w71) -> (w70:T19)  [unwired: 1 in]
                n30 = Unbundle By Name(w78) -> ("Self Reference"=w77:refnum<class "Lockin.DAQ.lvclass">)
                n31 = local write "Method"("setAIconfig" ("String")) -> ()
                n32 = local write "Payload"(w70) -> ()
                n33 = call "Write AI Configuration.vi"("error in (no error)"=w76, "AI Configuration"=w72, "Lockin.DAQ"=w77) -> ("error out"=w75:errorcluster, "Lockin.DAQ out"=w74:refnum<class "Lockin.DAQ.lvclass">)  [unwired: 7 in]
                n34 = Bundle By Name(cluster=w74, "Simulation mode"=w71) -> (w73:refnum<class "Lockin.DAQ.lvclass">)
                n35 = Bundle By Name(cluster=w78, "Self Reference"=w73) -> (w80:T13)
                n36 = call <vilib>:"Add State(s) to Queue__jki_lib_state_machine.vi"("State(s) in (\"\")"=w82) -> ("States Out"=w81:string)  [unwired: 14 in]
              }
              event User Event {
                n37 = event-data() -> ("AO Channels"=w83:T20)  [unwired: 1 in]
                n38 = local write "Payload"(w83) -> ()
                n39 = Unbundle By Name(w88) -> ("Self Reference"=w86:refnum<class "Lockin.DAQ.lvclass">)
                n40 = local write "Method"("setAO" ("String")) -> ()
                n41 = call "Write Channels_ AO.vi"("error in (no error)"=w85, "Channels: AO"=w83, "Lockin.DAQ"=w86) -> ("error out"=w84:errorcluster, "Lockin.DAQ out"=w87:refnum<class "Lockin.DAQ.lvclass">)  [unwired: 7 in]
                n42 = Bundle By Name(cluster=w88, "Self Reference"=w87) -> (w90:T13)
                n43 = call <vilib>:"Add State(s) to Queue__jki_lib_state_machine.vi"("State(s) in (\"\")"=w92) -> ("States Out"=w91:string)  [unwired: 14 in]
              }
              event User Event {
                n44 = event-data() -> ("AI Channels"=w94:T23)  [unwired: 1 in]
                n45 = local write "Payload"(w94) -> ()
                n46 = Unbundle By Name(w97) -> ("Self Reference"=w96:refnum<class "Lockin.DAQ.lvclass">)
                n47 = local write "Method"("setAI" ("String")) -> ()
                n48 = Bundle By Name(cluster=w96, "AI Channels"=w94) -> (w95:refnum<class "Lockin.DAQ.lvclass">)
                n49 = Bundle By Name(cluster=w97, "Self Reference"=w95) -> (w99:T13)
                n50 = call <vilib>:"Add State(s) to Queue__jki_lib_state_machine.vi"("State(s) in (\"\")"=w101) -> ("States Out"=w100:string)  [unwired: 14 in]
              }
              event User Event {
                n51 = event-data() -> ("REF Channels"=w102:T25)  [unwired: 1 in]
                n52 = local write "Method"("setREF" ("String")) -> ()
                n53 = local write "Payload"(w102) -> ()
                n54 = Unbundle By Name(w107) -> ("Self Reference"=w106:refnum<class "Lockin.DAQ.lvclass">)
                n55 = call "Write Channels_ Reference.vi"("error in (no error)"=w104, "Configuration.Channels: REF"=w102, "Lockin.DAQ"=w106) -> ("error out"=w103:errorcluster, "Lockin.DAQ out"=w105:refnum<class "Lockin.DAQ.lvclass">)  [unwired: 7 in]
                n56 = Bundle By Name(cluster=w107, "Self Reference"=w105) -> (w109:T13)
                n57 = call <vilib>:"Add State(s) to Queue__jki_lib_state_machine.vi"("State(s) in (\"\")"=w111) -> ("States Out"=w110:string)  [unwired: 14 in]
              }
              event User Event {
                n58 = event-data() -> ("setGain"=w112:T27)  [unwired: 1 in]
                n59 = local write "Method"("setInputGain" ("String")) -> ()
                n60 = Unbundle By Name(w117) -> ("Self Reference"=w116:refnum<class "Lockin.DAQ.lvclass">)
                n61 = local write "Payload"(w112) -> ()
                n62 = call "Write Gain.vi"("error in (no error)"=w115, "Input Gain"=w112, "Lockin.DAQ"=w116) -> ("error out"=w114:errorcluster, "Lockin.DAQ out"=w113:refnum<class "Lockin.DAQ.lvclass">)  [unwired: 7 in]
                n63 = Bundle By Name(cluster=w117, "Self Reference"=w113) -> (w119:T13)
                n64 = call <vilib>:"Add State(s) to Queue__jki_lib_state_machine.vi"("State(s) in (\"\")"=w121) -> ("States Out"=w120:string)  [unwired: 14 in]
              }
              event User Event {
                n65 = event-data() -> ("setGain"=w122:T27)  [unwired: 1 in]
                n66 = local write "Method"("setOutputGain" ("String")) -> ()
                n67 = Unbundle By Name(w126) -> ("Self Reference"=w124:refnum<class "Lockin.DAQ.lvclass">)
                n68 = Bundle By Name(cluster=w124, "Output Gain"=w122) -> (w123:refnum<class "Lockin.DAQ.lvclass">)
                n69 = local write "Payload"(w122) -> ()
                n70 = Bundle By Name(cluster=w126, "Self Reference"=w123) -> (w128:T13)
                n71 = call <vilib>:"Add State(s) to Queue__jki_lib_state_machine.vi"("State(s) in (\"\")"=w130) -> ("States Out"=w129:string)  [unwired: 14 in]
              }
              event User Event {
                n72 = event-data() -> ("Sampling"=w137:T28, "Sample Mode"=w136:T7, "AI Buffer Size (S)"=w135:i32, "Decimation"=w131:i32)  [unwired: 1 in]
                n73 = Unbundle By Name(w145) -> ("Self Reference"=w144:refnum<class "Lockin.DAQ.lvclass">)
                n74 = local write "Method"("setSampling" ("String")) -> ()
                n75 = Bundle("Sampling"=w137, "Sample Mode"=w136, "AI Buffer Size (S)"=w135, "Decimation"=w131) -> (w134:T29)  [unwired: 1 in]
                n76 = call "Write sampling.vi"("error in (no error)"=w141, "sampling"=w137, "Lockin.DAQ"=w144) -> ("error out"=w142:errorcluster, "Lockin.DAQ out"=w143:refnum<class "Lockin.DAQ.lvclass">)  [unwired: 7 in]
                n77 = local write "Payload"(w134) -> ()
                n78 = call "Write sample mode.vi"("error in (no error)"=w142, "sample mode"=w136, "Lockin.DAQ"=w143) -> ("error out"=w139:errorcluster, "Lockin.DAQ out"=w140:refnum<class "Lockin.DAQ.lvclass">)  [unwired: 7 in]
                n79 = call "Write buffer size (S).vi"("error in (no error)"=w139, "buffer size (S)"=w135, "Lockin.DAQ"=w140) -> ("error out"=w138:errorcluster, "Lockin.DAQ out"=w133:refnum<class "Lockin.DAQ.lvclass">)  [unwired: 7 in]
                n80 = Bundle By Name(cluster=w133, "decimation"=w131) -> (w132:refnum<class "Lockin.DAQ.lvclass">)
                n81 = Bundle By Name(cluster=w145, "Self Reference"=w132, "sample mode"=w136) -> (w147:T13)
                n82 = call <vilib>:"Add State(s) to Queue__jki_lib_state_machine.vi"("State(s) in (\"\")"=w149) -> ("States Out"=w148:string)  [unwired: 14 in]
              }
              event User Event {
                n83 = event-data() -> ("setSweep"=w151:T30)  [unwired: 1 in]
                n84 = Unbundle By Name(w154) -> ("Self Reference"=w153:refnum<class "Lockin.DAQ.lvclass">)
                n85 = Bundle By Name(cluster=w153, "Sweep Configuration"=w151) -> (w152:refnum<class "Lockin.DAQ.lvclass">)
                n86 = Bundle By Name(cluster=w154, "Self Reference"=w152) -> (w156:T13)
                n87 = call <vilib>:"Add State(s) to Queue__jki_lib_state_machine.vi"("State(s) in Front (\"\")"="" ("State(s) in Front (\"\")"), "State(s) in (\"\")"=w158) -> ("States Out"=w157:string)  [unwired: 13 in]
              }
              event User Event {
                n88 = event-data() -> ("measureOffset"=w159:T33)  [unwired: 1 in]
                n89 = local write "measure offset"(w159) -> ()
                n90 = Bundle By Name(cluster=w161, "Measure Offset"=w159) -> (w160:T13)
                n91 = call <vilib>:"Add State(s) to Queue__jki_lib_state_machine.vi"("State(s) in Front (\"\")"="DSP: Measure DAQ Offset" ("State(s) in Front (\"\")"), "State(s) in (\"\")"=w165) -> ("States Out"=w164:string)  [unwired: 13 in]
              }
              event User Event {
                n92 = event-data() -> ("Reset Phase"=w166:T34)  [unwired: 1 in]
                n93 = Bundle By Name(cluster=w168, "Reset Phase"=w166) -> (w167:T13)
                n94 = local write "Reset Phase?"(w166) -> ()
                n95 = call <vilib>:"Add State(s) to Queue__jki_lib_state_machine.vi"("State(s) in (\"\")"=w171) -> ("States Out"=w170:string)  [unwired: 14 in]
              }
              event User Event {
                n96 = event-data() -> ()  [unwired: 1 in, 5 out]
                n97 = call <vilib>:"Add State(s) to Queue__jki_lib_state_machine.vi"("State(s) in Front (\"\")"="DAQ: AUTO" ("State(s) in Front (\"\")"), "State(s) in (\"\")"=w176) -> ("States Out"=w175:string)  [unwired: 13 in]
              }
              event User Event {
                n98 = event-data() -> ("PreFilter"=w180:T35)  [unwired: 1 in, 4 out]
                n99 = Unbundle By Name(w180) -> ("60 Hz prefilter"=w179:bool, "LP prefilter"=w178:bool, "LP cutoff (Hz)"=w177:dbl)
                n100 = local write "60 Hz Prefilter?"(w179) -> ()
                n101 = local write "LP filter?"(w178) -> ()
                n102 = local write "LP Cutoff (Hz)"(w177) -> ()
                n103 = call <vilib>:"Add State(s) to Queue__jki_lib_state_machine.vi"("State(s) in Front (\"\")"="" ("State(s) in Front (\"\")"), "State(s) in (\"\")"=w185) -> ("States Out"=w184:string)  [unwired: 13 in]
              }
              event User Event {
                n104 = event-data() -> ()  [unwired: 1 in, 1 out]
                n105 = local write "zero offset"(TRUE ("zero offset")) -> ()
                n106 = call <vilib>:"Add State(s) to Queue__jki_lib_state_machine.vi"("State(s) in Front (\"\")"="DSP: Zero DAQ Offset" ("State(s) in Front (\"\")"), "State(s) in (\"\")"=w191) -> ("States Out"=w190:string)  [unwired: 13 in]
              }
              event User Event {
                # "example API call order:\ncontinuous acquisiton:\nsetAOconfig\nsetAIconfig\nsetSampling\nsetAO\nsetAI\nsetState start\n\nsetAO\nsetAO\nsetAO\n\nsetAOconfig\nsetState reset"
                # "start: Start acquisition (Macro: Acquire)\nstop: Stop acquisition (Macro: Stop)\nreset: Stop and Start acquisition (Macro: Stop, Macro: Start)\n\nif already running:\n- the private events setAOconfig, setAIconfig, setSampling\nwill be written to data cluster, but otherwise will be ignored until\nacquisition is reset\n- setAO and setREF will be implemented on next Acquisition iteration"
                n107 = event-data() -> ("setState"=w194:T36)  [unwired: 1 in, 4 out]
                n108 = local write "Payload"(w194) -> ()
                n109 = local write "Method"("setState" ("String")) -> ()
                n110 = Unbundle By Name(w193) -> ("state"=w195:T1)
                n111 = case shown="\"reset\"" w194 {
                  tunnel: ["Macro: Acquire" ("State(s) in Front (\"\")") "Macro: Stop" ("State(s) in Front (\"\")") "Macro: Stop\nMacro: Acquire" ("State(s) in Front (\"\")") w211 "" ("State(s) in Front (\"\")")] -> w196
                  tunnel: w195 -> [_ _ _ w209 _]
                  tunnel: w193 -> [w201 w203 w208 w213 w219]
                  tunnel: [w201 w203 w207 w212 w218] -> w192
                  frame "start", Default {
                  }
                  frame "stop" {
                  }
                  frame "reset" {
                    n112 = Bundle By Name(cluster=w208, "sweep index"=4) -> (w207:T13)
                  }
                  frame "start sweep" {
                    n113 = case shown="Default" w209 {
                      tunnel: ["Macro: Acquire" ("State(s) in Front (\"\")") "" ("State(s) in Front (\"\")")] -> w211
                      frame "idle", "stopped" {
                      }
                      frame Default {
                      }
                    }
                    n114 = Bundle By Name(cluster=w213, "sweep index"=0) -> (w212:T13)
                  }
                  frame "stop sweep" {
                    n115 = Bundle By Name(cluster=w219, "sweep index"=4) -> (w218:T13)
                  }
                }
                n116 = call <vilib>:"Add State(s) to Queue__jki_lib_state_machine.vi"("State(s) in (\"\")"=w200, "State(s) at Back (\"\")"=w196) -> ("States Out"=w199:string)  [unwired: 13 in]
              }
              event User Event {
                # "check calibration"
                # "calibrate"
                n117 = event-data() -> ("setCalibration"=w224:T37)  [unwired: 1 in, 4 out]
                n118 = local write "Method"("setCalibration" ("String")) -> ()
                n119 = local write "Payload"(w224) -> ()
                n120 = Select(t="True", s=w224, f="False" ("Arguments (\"\")")) -> (s? t:f=w221:string)
                n121 = call <vilib>:"Build State String with Arguments__JKI_lib_State_Machine.vi"("Arguments (\"\")"=w221, "State"="DAQ: CALIBRATE" ("State(s) in Front (\"\")")) -> ("State with Arguments"=w226:string)  [unwired: 4 in]
                n122 = call <vilib>:"Add State(s) to Queue__jki_lib_state_machine.vi"("State(s) in (\"\")"=w230, "State(s) at Back (\"\")"=w226) -> ("States Out"=w229:string)  [unwired: 13 in]
              }
              event Panel Close? {
                # "Discard the event because we'll close the front panel ourselves in Macro: Exit"
                # "Close Panel button (pressed) Event\n(this executes Macro: Exit to terminate the VI)"
                n123 = event-data() -> ()  [unwired: 1 in, 1 out]
                n124 = event-data("Discard?"=FALSE) -> ()  [unwired: 1 in, 1 out]
                n125 = call <vilib>:"Add State(s) to Queue__jki_lib_state_machine.vi"("State(s) in Front (\"\")"="//Macro: Exit", "State(s) in (\"\")"=w236) -> ("States Out"=w235:string)  [unwired: 13 in]
              }
              event User Event {
                n126 = event-data() -> ()  [unwired: 1 in, 5 out]
                n127 = call <vilib>:"Add State(s) to Queue__jki_lib_state_machine.vi"("State(s) in Front (\"\")"="Macro: Exit", "State(s) in (\"\")"=w241) -> ("States Out"=w240:string)  [unwired: 13 in]
              }
              event User Event {
                # "On Abort, no nice macro exit, but exit right away"
                n128 = event-data() -> ()  [unwired: 1 in, 5 out]
                n129 = call <vilib>:"Add State(s) to Queue__jki_lib_state_machine.vi"("State(s) in Front (\"\")"="Exit", "State(s) in (\"\")"=w246) -> ("States Out"=w245:string)  [unwired: 13 in]
              }
            }
          }
          frame "---------- Core ----------" {
            # "Do not put any code in this frame.\n(it is a separator no-op)"
            n130 = call <vilib>:"Add State(s) to Queue__jki_lib_state_machine.vi"("State(s) in (\"\")"=w251) -> ("States Out"=w250:string)  [unwired: 14 in]
          }
          frame Default {
            w262 = 42 items=["No error", "Argument error", "Memory is full", "Out of zone", "End of file", "File already open", "Generic file I/O error", "File not found", "File permission error", "Disk is full", "Duplicate path", "Too many files open", "System feature not enabled", "Resource file not found", "Cannot add resource", "Resource not found", "Image not found", "Image memory error", "Pen does not exist", "Config type invalid", "Config token not found", "Config parse error", "Config memory error", "Bad external code format", "Bad external code offset", "External code not present", "Null window", "Destroy window error", "Null menu", "Print aborted", "Bad print record", "Print driver error", "Windows error during printing", "Memory error during printing", "Print dialog error", "Generic print error", "Invalid device refnum", "Device not found", "Device parameter error", "Device unit error", "Cannot open device", "Device call aborted", "Generic error", "Cancelled by user", "Object ID too low", "Object ID too high", "Object not in heap", "Unknown heap", "Unknown object (invalid DefProc)", "Unknown object (DefProc not in table)", "Message out of range", "Invalid (null) method", "Unknown message", "Manager call not supported", "Bad address", "Network operation in progress", "Network operation timed out", "Connection is busy", "Network attribute not supported", "Network error", "Address in use", "System out of memory", "Connection aborted", "Connection refused", "Not connected", "Already connected", "Connection closed", "Initialization error (interapplication manager)", "Bad occurrence", "Wait on unbound occurrence handler", "Occurrence queue overflow", "Datalog type conflict", "Unused", "Unrecognized type (interapplication manager)", "Memory corrupt", "Failed to make temporary DLL", "Old CIN version", "Drag socket not found", "Failed to load drop-object", "Failed to register OLE object", "Failed to release OLE object", "Format specifier type mismatch", "Unknown format specifier", "Too few format specifiers", "Too many format specifiers", "Scan failed", "Newer CIN version", "Error converting to variant", "Runtime menu error", "Password tampered", "Variant attribute not found", "Incompatible variant data type", "Event data is not available", "Event Store is not present", "Occurrence is not found", "Event Queue is not created", "Event info is not available", "Refnum passed is NULL", "Error retrieving Class GUID", "Error retrieving CoClass GUID", "Error retrieving TypeLib GUID.", "Bad built application magic bytes.", "Specific driver is different from the specific driver associated with the Logical Name.", "There is no session opened to the class driver.", "Max Error", "MAX - Error with config objects", "MAX - Error loading configuration", "MAX - Group not supported"]
            # "Current State"
            # "Do not delete, rename, or modify this frame.\n(this is used to capture unhandled states and typos)"
            # "Handle mistyped state name (developer tool)"
            n131 = Format Into String(format string="Software Exception: Unhandled State \"%s\"." ("message"), error in=w258, w253) -> (resulting string=w261:string, error out=w260:errorcluster)  [unwired: 1 in]
            n132 = call <vilib>:"Error Cluster From Error Code.vi"("show call chain? (False)"=TRUE, "error in (no error)"=w260, "error message (\"\")"=w261, "error code (0)"=w262) -> ("error out"=w259:errorcluster)  [unwired: 5 in]
            n133 = call <vilib>:"Add State(s) to Queue__jki_lib_state_machine.vi"("State(s) in (\"\")"=w257) -> ("States Out"=w256:string)  [unwired: 14 in]
          }
          frame "Initialize Core Data" {
            # "Do not delete, rename, or modify this frame.\n(this is used to determine panel behavior on exit)"
            # "originally closed?"
            # "exe?"
            # "If panel starts closed or is an EXE, then close it when we exit"
            n134 = property class="VI"() -> ("Front Panel.Open"=w272:bool)  [unwired: 2 in, 2 out]
            n135 = property class="App"() -> ("App.Kind"=w271:T3)  [unwired: 2 in, 2 out]
            n136 = control-ref of="Current VI Reference"() -> (w265:refnum<vi>)
            n137 = Not(x=w272) -> (.not. x?=w269:bool)
            n138 = Equal?(x=w271, y=T3."Run Time System" ("Application:Kind")) -> (x = y?=w268:bool)
            n139 = Or(x=w269, y=w268) -> (x .or. y?=w266:bool)
            n140 = Bundle By Name(cluster=w267, "Core.Current VI Reference"=w265, "Core.Close Panel on Exit?"=w266) -> (w274:T13)
            n141 = call <vilib>:"Add State(s) to Queue__jki_lib_state_machine.vi"("State(s) in (\"\")"=w276) -> ("States Out"=w275:string)  [unwired: 14 in]
          }
          frame "Error Handler" {
            w290 = FALSE  # Stop on Unhandled Error (T)
            w296 = errorcluster {"status"=FALSE, "code"=0, "source"=""}  # No error
            # "if there are two subsequent errors that are the same, don't retry"
            # "Overwrite this method to handle errors and pass to parent if not handled. Parent will fire a public event if the error is not handled up the chain of classes."
            n142 = Unbundle By Name(w295) -> ("Core.error.code"=w279:i32, "Self Reference"=w288:refnum<class "Lockin.DAQ.lvclass">)
            n143 = call "Lockin.DAQ.ErrorHandler.vi"("error in (no error)"=w278, "Lockin.DAQ in"=w288) -> ("error out"=w289:errorcluster, "Error Filtered?"=w286:bool, "Lockin.DAQ out"=w287:refnum<class "Lockin.DAQ.lvclass">)  [unwired: 6 in, 1 out]
            n144 = Unbundle By Name(w278) -> ("code"=w277:i32)
            n145 = call-dynamic "Handle Error.vi"("Stop on Unhandled Error (T)"=w290, "error in"=w289, "SMO"=w287) -> ("handling error"=w291:errorcluster)  [unwired: 6 in, 2 out]
            n146 = Equal?(x=w279, y=w277) -> (x = y?=w280:bool)
            n147 = Bundle By Name(cluster=w295, "Core.error"=w278) -> (w294:T13)
            n148 = Select(t="Exit", s=w291, f="") -> (s? t:f=w284:string)
            n149 = Select(t="", s=w280, f="\nDAQ: STOP\nDAQ: CLEAR\nMacro: Acquire" ("States Out")) -> (s? t:f=w282:string)
            n150 = Select(t=w282, s=w286, f=w284) -> (s? t:f=w285:string)
          }
          frame "Exit" {
            # "Do not put any code in this frame.\n(No errors that occur here will be handled.)"
            n151 = Unbundle By Name(w299) -> ("Core.error"=w298:errorcluster)
            n152 = call <vilib>:"Add State(s) to Queue__jki_lib_state_machine.vi"("State(s) in (\"\")"=w303) -> ("States Out"=w302:string)  [unwired: 14 in]
          }
          frame "---------- Data ----------" {
            # "Do not put any code in this frame.\n(It is a separator no-op. You can make a copy of this frame to create a new Data frame)"
            n153 = call <vilib>:"Add State(s) to Queue__jki_lib_state_machine.vi"("State(s) in (\"\")"=w308) -> ("States Out"=w307:string)  [unwired: 14 in]
          }
          frame "Data: Initialize" {
            w309 = FALSE  # Measure Offset
            w310 = FALSE  # Reset Phase
            w311 = T38 {"X"=[], "Y"=[]}  # Reference
            w313 = waveform(dbl)[] []  # Sweep_AO
            w312 = waveform(dbl)[] []  # Sweep_AI
            (unwired) T39 {"Sweep_AO"=[], "Sweep_AI"=[]}  # IVSweepResults []
            w314 = dbl[] []  # DAQ Offset
            w315 = T6 {"X results"=[], "Y Results"=[]}  # SweepResults []
            w316 = T6 {"X results"=[], "Y Results"=[]}  # SweepResults [i]
            w317 = -1  # sweep index
            w318 = T7 10178 items=["Finite Samples"=10178, "Continuous Samples"=10123]  # sample mode
            w323 = T12 {"Time Stamp"=timestamp(0 s since 1904-01-01), "Results"=[]}  # Results
            w322 = State-enum."idle"  # state
            w325 = -1  # to
            w327 = waveform(dbl)[] []  # AO
            w326 = waveform(dbl)[] []  # AI
            w328 = T40 {"Current VI Reference"=refnum, "Close Panel on Exit?"=FALSE, "error"={"status"=FALSE, "code"=0, "source"=""}}  # Core
            w331 = refnum<class "Lockin.DAQ.lvclass"> refnum  # Self Reference
            # "start in idle mode"
            # "do not delete - used by framework"
            # "Data names and types of shift register data are defined by this bundle."
            # "Initialize the shift-register data, here.\n(data names are defined by what you wire into the bundle function)"
            n154 = Variant To Data(error in=w332, type=w331, Variant=w330) -> (data=w321:refnum<class "Lockin.DAQ.lvclass">, error out=w320:errorcluster)
            n155 = call "Lockin.DAQ.getDAQState.vi"("error in (no error)"=w320, "state"=w322, "Lockin.DAQ"=w321) -> ("error out"=w319:errorcluster)  [unwired: 7 in, 1 out]
            n156 = local write "DAQ state"(w322) -> ()
            n157 = call <vilib>:"Add State(s) to Queue__jki_lib_state_machine.vi"("State(s) in (\"\")"=w334) -> ("States Out"=w333:string)  [unwired: 14 in]
            n158 = Bundle("Core"=w328, "Self Reference"=w321, "to"=w325, "state"=w322, "sample mode"=w318, "AO"=w327, "AI"=w326, "Reference"=w311, "Results"=w323, "sweep index"=w317, "SweepResults [i]"=w316, "SweepResults []"=w315, "DAQ Offset"=w314, "Sweep_AO"=w313, "Sweep_AI"=w312, "Reset Phase"=w310, "Measure Offset"=w309) -> (w324:T13)  [unwired: 1 in]
          }
          frame "Data: Cleanup" {
            # "Cleanup any data and references, here.\n(this is called automatically, by the Macro: Exit)"
            n159 = Unbundle By Name(w335) -> ("Core.Current VI Reference"=w339:refnum<vi>)
            n160 = Close Reference(reference=w339, error in (no error)=w338) -> (error out=w337:errorcluster)
            n161 = call <vilib>:"Add State(s) to Queue__jki_lib_state_machine.vi"("State(s) in (\"\")"=w341) -> ("States Out"=w340:string)  [unwired: 14 in]
          }
          frame "---------- UI ----------" {
            # "Do not put any code in this frame.\n(It is a separator no-op. You can make a copy of this frame to create a new UI frame)"
            n162 = call <vilib>:"Add State(s) to Queue__jki_lib_state_machine.vi"("State(s) in (\"\")"=w346) -> ("States Out"=w345:string)  [unwired: 14 in]
          }
          frame "UI: Initialize" {
            # "Initialize the User Interface, here.\n(this is called automatically, by the Macro: Init)"
            n163 = local write "Method"("" ("String")) -> ()
            n164 = call <vilib>:"Add State(s) to Queue__jki_lib_state_machine.vi"("State(s) in (\"\")"=w352) -> ("States Out"=w351:string)  [unwired: 14 in]
          }
          frame "UI: Cursor Set" {
            # "Argument"
            # "Initialize the User Interface, here.\n(this is called automatically, by the Macro: Init)"
            n165 = disable-structure shown="Default" {
              disable-tunnel: w355 -> [w360 w363]
              disable-tunnel: [w360 w362] -> w354
              disable-tunnel: w353 -> [_ w361]
              frame condition #0 {
              }
              frame condition #1 (active) {
                n166 = case shown="\"Idle\", Default" w361 {
                  tunnel: w363 -> [w365 w367]
                  tunnel: [w364 w366] -> w362
                  frame "Idle", Default {
                    n167 = call <vilib>:"Unset Busy.vi"("error in (no error)"=w365) -> ("error out"=w364:errorcluster)  [unwired: 10 in]
                  }
                  frame "Busy" {
                    n168 = call <vilib>:"Set Busy.vi"("error in (no error)"=w367) -> ("error out"=w366:errorcluster)  [unwired: 9 in, 1 out]
                  }
                }
              }
            }
            n169 = call <vilib>:"Add State(s) to Queue__jki_lib_state_machine.vi"("State(s) in (\"\")"=w359) -> ("States Out"=w358:string)  [unwired: 14 in]
          }
          frame "UI: Front Panel State" {
            # "Argument"
            # "Set Front Panel Open or Closed\n(Usage: \"UI: Front Panel State >> Open|Close\")"
            n170 = Unbundle By Name(w371) -> ("Core.Current VI Reference"=w370:refnum<vi>)
            n171 = disable-structure shown="Default" {
              disable-tunnel: w373 -> [w379 w402]
              disable-tunnel: [w378 w402] -> w372
              disable-tunnel: w370 -> [w377 _]
              disable-tunnel: w369 -> [w376 _]
              frame condition #0 (active) {
                n172 = case shown="\"Close\"" w376 {
                  tunnel: w379 -> [w383 w396]
                  tunnel: [w385 w397] -> w378
                  tunnel: w377 -> [w384 w394]
                  frame "Open", Default {
                    n173 = property class="VI"(reference=w384, error in=w383) -> (reference out=w381:refnum<vi>, error out=w382:errorcluster, "FP.State"=w380:T4)
                    n174 = case shown="\"Closed\"" w380 {
                      tunnel: [w388 w391] -> w385
                      tunnel: w382 -> [w387 w391]
                      tunnel: w381 -> [w386 _]
                      frame "Closed" {
                        n175 = invoke class="VI" method="FP.Open"(reference=w386, error in=w387, "Activate"=TRUE, "State"=T4."Standard") -> (error out=w388:errorcluster)  [unwired: 1 in, 4 out]
                      }
                      frame Default {
                      }
                    }
                  }
                  frame "Close" {
                    n176 = property class="VI"(reference=w394, error in=w396) -> (reference out=w393:refnum<vi>, error out=w395:errorcluster, "FP.State"=w392:T4)
                    n177 = case shown="Default" w392 {
                      tunnel: [w398 w401] -> w397
                      tunnel: w395 -> [w398 w400]
                      tunnel: w393 -> [_ w399]
                      frame "Invalid", "Closed" {
                      }
                      frame Default {
                        n178 = invoke class="VI" method="FP.Close"(reference=w399, error in=w400) -> (error out=w401:errorcluster)  [unwired: 1 in, 2 out]
                      }
                    }
                  }
                }
              }
              frame condition #1 {
              }
            }
            n179 = call <vilib>:"Add State(s) to Queue__jki_lib_state_machine.vi"("State(s) in (\"\")"=w375) -> ("States Out"=w374:string)  [unwired: 14 in]
          }
          frame "---------- Macro ----------" {
            # "Do not put any code in this frame.\n(It is a separator no-op. You can make a copy of this frame to create a new Macro frame)"
            n180 = call <vilib>:"Add State(s) to Queue__jki_lib_state_machine.vi"("State(s) in (\"\")"=w407) -> ("States Out"=w406:string)  [unwired: 14 in]
          }
          frame "Macro: Initialize" {
            w412 = "UI: Initialize\nUI: Front Panel State >> Open"  # UI: Initialize UI: Front Panel State >> Open
            w408 = "Process: Sync"
            # "Initialization Macro\n(This is called once, when the VI starts)"
            n181 = control-ref of="This VI"() -> (w410:refnum<vi>)
            n182 = property class="VI"(reference=w410) -> ("Exec.State"=w409:T5)  [unwired: 1 in, 2 out]
            n183 = Equal?(x=w409, y=T5."Run top level") -> (x = y?=w415:bool)
            n184 = Select(t=w408, s=w415, f="") -> ()  [unwired: 1 out]
            n185 = call <vilib>:"Add State(s) to Queue__jki_lib_state_machine.vi"("State(s) in Front (\"\")"="Data: Initialize\nInitialize Core Data\nEvents: Register", "State(s) in (\"\")"=w408, "State(s) at Back (\"\")"=w412) -> ("States Out"=w411:string)  [unwired: 12 in]
            n186 = call <vilib>:"Add State(s) to Queue__jki_lib_state_machine.vi"("State(s) in Front (\"\")"=w411, "State(s) in (\"\")"=w421) -> ("States Out"=w420:string)  [unwired: 13 in]
          }
          frame "Macro: Exit" {
            # "Exit Macro\n(This is called once, when the VI exits)"
            n187 = Unbundle By Name(w428) -> ("Core.Close Panel on Exit?"=w433:bool)
            n188 = Select(t="UI: Front Panel State >> Close", s=w433, f="") -> (s? t:f=w430:string)
            n189 = call <vilib>:"Add State(s) to Queue__jki_lib_state_machine.vi"("State(s) in Front (\"\")"="\nData: Cleanup\nEvents: Unregister", "State(s) in (\"\")"="Process: Sync", "State(s) at Back (\"\")"="Exit") -> ("States Out"=w425:string)  [unwired: 12 in]
            n190 = call <vilib>:"Add State(s) to Queue__jki_lib_state_machine.vi"("State(s) in Front (\"\")"="Macro: Stop", "State(s) in (\"\")"=w430, "State(s) at Back (\"\")"=w425) -> ("States Out"=w423:string)  [unwired: 12 in]
            n191 = call <vilib>:"Add State(s) to Queue__jki_lib_state_machine.vi"("State(s) in Front (\"\")"=w423, "State(s) in (\"\")"=w436) -> ("States Out"=w435:string)  [unwired: 13 in]
          }
          frame "Macro: Acquire" {
            (unwired) "DAQ: TIMED LOOP\nDAQ: STOP\nDAQ: CLEAR" ("State(s) in Front (\"\")")
            w445 = 10178 items=["Finite Samples"=10178, "Continuous Samples"=10123] ("sample mode")
            # "#todo:\ndo not create/clear tasks every time"
            # "note (8/23/2019):\nCREATE/START & STOP/CLEAR go hand-in-hand in the macro, but they are separated to make it easier to add features (e.g. event registration b/w CREATE and START)"
            # "already running = \nDAQmx tasks are STARTED"
            n192 = Unbundle By Name(w444) -> ("state"=w438:T1, "sample mode"=w441:T7)
            n193 = Equal?(x=w441, y=w445) -> (x = y?=w440:bool)
            n194 = case shown="\"idle\", Default" w438 {
              tunnel: ["DAQ: CREATE\n//DAQ: Event\nDAQ: START" ("State(s) in Front (\"\")") "" ("State(s) in Front (\"\")")] -> w442
              frame "idle", Default {
              }
              frame "created" {
              }
            }
            n195 = case shown="True" w440 {
              tunnel: ["" ("State(s) in Front (\"\")") "DAQ: STOP\nDAQ: CLEAR" ("State(s) in Front (\"\")")] -> w439
              frame False {
              }
              frame True {
              }
            }
            n196 = call <vilib>:"Add State(s) to Queue__jki_lib_state_machine.vi"("State(s) in Front (\"\")"=w442, "State(s) in (\"\")"="Macro: Generate\nDAQ: AO AI\nMacro: DSP\nMacro: Sweep" ("State(s) in Front (\"\")"), "State(s) at Back (\"\")"=w439) -> ("States Out"=w443:string)  [unwired: 12 in]
            n197 = call <vilib>:"Add State(s) to Queue__jki_lib_state_machine.vi"("State(s) in Front (\"\")"=w443, "State(s) in (\"\")"=w449) -> ("States Out"=w448:string)  [unwired: 13 in]
          }
          frame "Macro: Generate" {
            # "Do not put any code in this frame.\n(It is a separator no-op. You can make a copy of this frame to create a new Macro frame)"
            n198 = call <vilib>:"Add State(s) to Queue__jki_lib_state_machine.vi"("State(s) in Front (\"\")"="Generate: Generate" ("State(s) in Front (\"\")"), "State(s) in (\"\")"=w459) -> ("States Out"=w458:string)  [unwired: 13 in]
          }
          frame "Macro: DSP" {
            # "Do not put any code in this frame.\n(It is a separator no-op. You can make a copy of this frame to create a new Macro frame)"
            n199 = call <vilib>:"Add State(s) to Queue__jki_lib_state_machine.vi"("State(s) in Front (\"\")"="DSP: Phase" ("State(s) in Front (\"\")"), "State(s) at Back (\"\")"="DSP: Filter\nDSP: Lockin" ("State(s) in Front (\"\")")) -> ("States Out"=w462:string)  [unwired: 13 in]
            n200 = call <vilib>:"Add State(s) to Queue__jki_lib_state_machine.vi"("State(s) in Front (\"\")"=w462, "State(s) in (\"\")"=w467) -> ("States Out"=w466:string)  [unwired: 13 in]
          }
          frame "Macro: Sweep" {
            n201 = Unbundle By Name(w472) -> ("Self Reference"=w471:refnum<class "Lockin.DAQ.lvclass">, "sweep index"=w470:i32)
            "sweep index" <- w470
            n202 = case shown="4" w470 {
              tunnel: ["" ("State(s) in Front (\"\")") "Sweep: Initialize\nSweep: Set Initial\nSweep: Wait" ("State(s) in Front (\"\")") "Sweep: Wait" ("State(s) in Front (\"\")") "Sweep: Configure Sweep" ("State(s) in Front (\"\")") "Sweep: Done Sweeping?\nSweep: Save" ("State(s) in Front (\"\")") "Sweep: Stop" ("State(s) in Front (\"\")")] -> w469
              tunnel: w471 -> [_ _ _ _ _ _]
              frame -1, Default {
              }
              frame 0 {
              }
              frame 1 {
              }
              frame 2 {
              }
              frame 3 {
              }
              frame 4 {
              }
            }
            n203 = call <vilib>:"Add State(s) to Queue__jki_lib_state_machine.vi"("State(s) in Front (\"\")"=w469, "State(s) in (\"\")"=w475) -> ("States Out"=w474:string)  [unwired: 13 in]
          }
          frame "Macro: Stop" {
            n204 = call <vilib>:"Add State(s) to Queue__jki_lib_state_machine.vi"("State(s) in Front (\"\")"="DAQ: STOP\nDAQ: CLEAR" ("State(s) in Front (\"\")"), "State(s) in (\"\")"=w487) -> ("States Out"=w483:string)  [unwired: 13 in]
          }
          frame "---------- Process ----------" {
            # "Template Separator\n(You can make a copy of, or modify, this frame)"
            n205 = call <vilib>:"Add State(s) to Queue__jki_lib_state_machine.vi"("State(s) in (\"\")"=w492) -> ("States Out"=w491:string)  [unwired: 14 in]
          }
          frame "Process: Sync" {
            n206 = Unbundle By Name(w500) -> ("Self Reference"=w496:refnum<class "Lockin.DAQ.lvclass">)
            n207 = call <vilib>:"WaitOnProcessSync.vi"("error in (no error)"=w495, "SMO"=w496) -> ("error out"=w494:errorcluster, "Don't run?"=w499:bool)  [unwired: 7 in, 1 out]
            n208 = Select(t="Data: Cleanup\nEvents: Unregister\nExit", s=w499, f="") -> (s? t:f=w493:string)
            n209 = call <vilib>:"Add State(s) to Queue__jki_lib_state_machine.vi"("State(s) in Front (\"\")"=w493, "State(s) in (\"\")"=w503) -> ("States Out"=w502:string)  [unwired: 13 in]
          }
          frame "---------- Events ----------" {
            # "Template Separator\n(You can make a copy of, or modify, this frame)"
            n210 = call <vilib>:"Add State(s) to Queue__jki_lib_state_machine.vi"("State(s) in (\"\")"=w508) -> ("States Out"=w507:string)  [unwired: 14 in]
          }
          frame "Events: Register" {
            w509 = refnum<event-registration> refnum  # DAQmx
            w517 = refnum<event-registration> refnum  # SMO
            w518 = refnum<event-registration> refnum  # LockinDAQ
            # "Replace later"
            # "Expand to add\nmore events"
            n211 = Unbundle By Name(w529) -> ("Self Reference"=w528:refnum<class "Lockin.DAQ.lvclass">)
            n212 = call <vilib>:"GetProtectedEvents.vi"("SMO"=w528) -> ("error out"=w525:errorcluster, "SMO Protected Events"=w521:T41, "SMO out"=w524:refnum<class "Lockin.DAQ.lvclass">)  [unwired: 8 in]
            n213 = call "Lockin.DAQ.GetPrivateEvents.vi"("Lockin.DAQ"=w524) -> ("error out"=w511:errorcluster, "Private Events"=w520:T42)  [unwired: 8 in, 1 out]
            n214 = register-events(w521) -> (reference out=w523:refnum<event-registration>, error out=w516:errorcluster)  [unwired: 2 in]
            n215 = register-events(w520) -> (reference out=w519:refnum<event-registration>, error out=w513:errorcluster)  [unwired: 2 in]
            n216 = Variant To Data(error in=w513, type=w518, Variant=w519) -> (data=w510:refnum<event-registration>, error out=w514:errorcluster)
            n217 = Variant To Data(error in=w516, type=w517, Variant=w523) -> (data=w512:refnum<event-registration>, error out=w515:errorcluster)
            n218 = Bundle("SMO"=w512, "LockinDAQ"=w510, "DAQmx"=w509) -> (w522:T43)  [unwired: 1 in]
            n219 = Merge Errors(w515, w514, w511, w527, w525) -> (w526:errorcluster)
            n220 = call <vilib>:"Add State(s) to Queue__jki_lib_state_machine.vi"("State(s) in (\"\")"=w531) -> ("States Out"=w530:string)  [unwired: 14 in]
          }
          frame "Events: Unregister" {
            n221 = Unregister For Events(event registration refnum=w532, error in=w534) -> (error out=w533:errorcluster)
            n222 = call <vilib>:"Clear Errors.vi"("error in (no error)"=w533) -> ()  [unwired: 5 in, 2 out]
            n223 = call <vilib>:"Add State(s) to Queue__jki_lib_state_machine.vi"("State(s) in (\"\")"=w537) -> ("States Out"=w536:string)  [unwired: 14 in]
          }
          frame "---------- DAQ ----------" {
            n224 = call <vilib>:"Add State(s) to Queue__jki_lib_state_machine.vi"("State(s) in (\"\")"=w542) -> ("States Out"=w541:string)  [unwired: 14 in]
          }
          frame "DAQ: CREATE" {
            n225 = Unbundle By Name(w556) -> ("Self Reference"=w554:refnum<class "Lockin.DAQ.lvclass">, "state"=w544:T1)
            n226 = call <userlib>:"Tick Count (ms)__ogtk.vi"("error in (no error)"=w553) -> ("error out"=w547:errorcluster, "millisecond timer value"=w550:u32)  [unwired: 9 in]
            n227 = case shown="\"idle\"" w544 {
              selector: w544 -> [w563 _]
              tunnel: w554 -> [w562 w573]
              tunnel: [w562 w566] -> w548
              tunnel: w547 -> [w561 w572]
              tunnel: [w561 w567] -> w546
              tunnel: [w563 w565] -> w545
              tunnel: ["" ("State(s) in Front (\"\")") w564] -> w543
              frame Default {
              }
              frame "idle" {
                # "create DAQ tasks"
                n228 = call "Lockin.DAQ.Create.vi"("error in"=w572, "Lockin.DAQ"=w573) -> ("error out"=w569:errorcluster, "Lockin.DAQ"=w568:refnum<class "Lockin.DAQ.lvclass">)  [unwired: 8 in]
                n229 = case shown="No Error" w569 {
                  selector: w569 -> [w576 w580]
                  tunnel: [State-enum."created" ("state") State-enum."idle" ("state")] -> w565
                  tunnel: [w576 w580] -> w570
                  tunnel: w568 -> [w575 w579]
                  tunnel: [w575 w579] -> w571
                  tunnel: ["" ("State(s) in Front (\"\")") "DAQ: CLEAR" ("State(s) in Front (\"\")")] -> w564
                  frame No Error {
                  }
                  frame Error {
                  }
                }
                n230 = call "Lockin.DAQ.getDAQState.vi"("error in (no error)"=w570, "state"=w565, "Lockin.DAQ"=w571) -> ("error out"=w567:errorcluster, "Lockin.DAQ"=w566:refnum<class "Lockin.DAQ.lvclass">)  [unwired: 7 in]
              }
            }
            n231 = Bundle By Name(cluster=w556, "Self Reference"=w548, "state"=w545) -> (w555:T13)
            n232 = local write "DAQ state"(w545) -> ()
            n233 = call <userlib>:"Tick Count (ms)__ogtk.vi"("error in (no error)"=w546) -> ("error out"=w552:errorcluster, "millisecond timer value"=w551:u32)  [unwired: 9 in]
            n234 = Subtract(x=w551, y=w550) -> (x-y=→"DAQ Create Tasks (ms)":u32)
            n235 = call <vilib>:"Add State(s) to Queue__jki_lib_state_machine.vi"("State(s) in Front (\"\")"=w543, "State(s) in (\"\")"=w559) -> ("States Out"=w558:string)  [unwired: 13 in]
          }
          frame "DAQ: AUTO" {
            n236 = Unbundle By Name(w588) -> ("Self Reference"=w590:refnum<class "Lockin.DAQ.lvclass">)
            n237 = call "Auto Configure DAQ.vi"("error in (no error)"=w589, "Lockin.DAQ"=w590) -> ("error out"=w583:errorcluster, "New Ch []"=w586:T44[], "Lockin.DAQ"=w585:refnum<class "Lockin.DAQ.lvclass">)  [unwired: 7 in]
            n238 = call "Lockin.DAQ.getDAQconfig.vi"("error in (no error)"=w583, "getDAQconfig"=w586, "Lockin.DAQ"=w585) -> ("error out"=w582:errorcluster, "Lockin.DAQ"=w584:refnum<class "Lockin.DAQ.lvclass">)  [unwired: 7 in]
            n239 = Bundle By Name(cluster=w588, "Self Reference"=w584) -> (w587:T13)
            n240 = call <vilib>:"Add State(s) to Queue__jki_lib_state_machine.vi"("State(s) in (\"\")"=w593) -> ("States Out"=w592:string)  [unwired: 14 in]
          }
          frame "DAQ: START" {
            n241 = Unbundle By Name(w608) -> ("to"=w594:i32, "Self Reference"=w606:refnum<class "Lockin.DAQ.lvclass">, "state"=w595:T1)
            n242 = call <userlib>:"Tick Count (ms)__ogtk.vi"("error in (no error)"=w605) -> ("error out"=w600:errorcluster, "millisecond timer value"=w602:u32)  [unwired: 9 in]
            n243 = case shown="Default" w595 {
              selector: w595 -> [_ w632]
              tunnel: w606 -> [w621 w631]
              tunnel: w600 -> [w617 w633]
              tunnel: [w616 w633] -> w599
              tunnel: [w614 w631] -> w598
              tunnel: [w613 w630] -> w597
              tunnel: [w612 w632] -> w596
              tunnel: w594 -> [_ w630]
              frame Default {
                n244 = call "Lockin.DAQ.Start.vi"("error in"=w617, "Lockin.DAQ in"=w621) -> ("error out"=w620:errorcluster, "Lockin.DAQ out"=w618:refnum<class "Lockin.DAQ.lvclass">)  [unwired: 8 in]
                n245 = case shown="No Error" w620 {
                  selector: w620 -> [w623 w627]
                  tunnel: [State-enum."started" ("state") State-enum."idle" ("state")] -> w612
                  tunnel: [1 -1] -> w613
                  tunnel: [w623 w627] -> w619
                  tunnel: w618 -> [w622 w626]
                  tunnel: [w622 w626] -> w615
                  frame No Error {
                  }
                  frame Error {
                  }
                }
                n246 = call "Lockin.DAQ.getDAQState.vi"("error in (no error)"=w619, "state"=w612, "Lockin.DAQ"=w615) -> ("error out"=w616:errorcluster, "Lockin.DAQ"=w614:refnum<class "Lockin.DAQ.lvclass">)  [unwired: 7 in]
              }
              frame "started", "sweeping" {
              }
            }
            "DAQ state" <- w596
            n247 = Bundle By Name(cluster=w608, "to"=w597, "Self Reference"=w598, "state"=w596) -> (w607:T13)
            n248 = call <userlib>:"Tick Count (ms)__ogtk.vi"("error in (no error)"=w599) -> ("error out"=w604:errorcluster, "millisecond timer value"=w603:u32)  [unwired: 9 in]
            n249 = Subtract(x=w603, y=w602) -> (x-y=→"DAQ Start Tasks (ms)":u32)
            n250 = call <vilib>:"Add State(s) to Queue__jki_lib_state_machine.vi"("State(s) in (\"\")"=w611) -> ("States Out"=w610:string)  [unwired: 14 in]
          }
          frame "DAQ: AO AI" {
            # "signal at device"
            # "signal at device"
            # "write AO\nread AI"
            n251 = Unbundle By Name(w647) -> ("Self Reference"=w644:refnum<class "Lockin.DAQ.lvclass">, "AO"=w643:waveform(dbl)[])
            n252 = call <userlib>:"Tick Count (ms)__ogtk.vi"("error in (no error)"=w645) -> ("error out"=w640:errorcluster, "millisecond timer value"=w637:u32)  [unwired: 9 in]
            n253 = call "Lockin.DAQ.Read AI and Write AO.vi"("error in (no error)"=w640, "AO []"=w643, "Lockin.DAQ in"=w644) -> ("error out"=w641:errorcluster, "AO []"=w634:waveform(dbl)[], "AI []"=w635:waveform(dbl)[], "Lockin.DAQ out"=w642:refnum<class "Lockin.DAQ.lvclass">)  [unwired: 5 in]
            n254 = Bundle By Name(cluster=w647, "Self Reference"=w642, "AI"=w635, "AO"=w634) -> (w646:T13)
            n255 = call <userlib>:"Tick Count (ms)__ogtk.vi"("error in (no error)"=w641) -> ("error out"=w639:errorcluster, "millisecond timer value"=w638:u32)  [unwired: 9 in]
            n256 = Subtract(x=w638, y=w637) -> (x-y=→"DAQ AO/AI (ms)":u32)
            n257 = call <vilib>:"Add State(s) to Queue__jki_lib_state_machine.vi"("State(s) in (\"\")"=w650) -> ("States Out"=w649:string)  [unwired: 14 in]
          }
          frame "DAQ: TIMED LOOP" {
            # "!!!!!!!!!!!!!!!!!!!!!!!!!!!!!!!!!!!!!!!!!!!!!!!!!!!!!!!!!!!!!!!!!!!!!!!!\nTHIS IS AN EXPERIMENTAL BLOCKING CALL TO:\nGenerate\nRead/Write\nDSP\nIt should listen to events that change AO or REF Channels.\nInside there is a timed loop that will not stop unless it receives events for Set State = stop; SMO Stop; or SMO error\n!!!!!!!!!!!!!!!!!!!!!!!!!!!!!!!!!!!!!!!!!!!!!!!!!!!!!!!!!!!!!!!!!!!!!"
            n258 = Unbundle By Name(w657) -> ("Self Reference"=w654:refnum<class "Lockin.DAQ.lvclass">)
            n259 = call "Lockin.DAQ.TimedLoop.vi"("error in (no error)"=w652, "Event Cluster"=w655, "Lockin.DAQ in"=w654) -> ("error out"=w651:errorcluster, "Lockin.DAQ out"=w653:refnum<class "Lockin.DAQ.lvclass">)  [unwired: 7 in]
            n260 = Bundle By Name(cluster=w657, "Self Reference"=w653) -> (w656:T13)
            n261 = call <vilib>:"Add State(s) to Queue__jki_lib_state_machine.vi"("State(s) in (\"\")"=w659) -> ("States Out"=w658:string)  [unwired: 14 in]
          }
          frame "DAQ: CALIBRATE" {
            # "calibrate or get calibration"
            n262 = Unbundle By Name(w669) -> ("Self Reference"=w666:refnum<class "Lockin.DAQ.lvclass">)
            n263 = case shown="\"False\", Default" w667 {
              tunnel: w666 -> [w677 w682]
              tunnel: [w676 w681] -> w662
              tunnel: w665 -> [w674 w680]
              tunnel: [w675 w679] -> w664
              tunnel: [w673 w678] -> w663
              frame "False", Default {
                n264 = call "Lockin.DAQ.Get Calibration.vi"("error in (no error)"=w674, "Lockin.DAQ in"=w677) -> ("error out"=w675:errorcluster, "Cal Info"=w673:T45[], "Lockin.DAQ out"=w676:refnum<class "Lockin.DAQ.lvclass">)  [unwired: 7 in]
              }
              frame "True" {
                n265 = call "Lockin.DAQ.Calibrate.vi"("error in (no error)"=w680, "Lockin.DAQ in"=w682) -> ("error out"=w679:errorcluster, "Cal Info"=w678:T45[], "Lockin.DAQ out"=w681:refnum<class "Lockin.DAQ.lvclass">)  [unwired: 7 in]
              }
            }
            n266 = call "Lockin.DAQ.getCalibration.vi"("error in (no error)"=w664, "getCalibration"=w663, "Lockin.DAQ"=w662) -> ("error out"=w660:errorcluster, "Lockin.DAQ"=w661:refnum<class "Lockin.DAQ.lvclass">)  [unwired: 7 in]
            n267 = Bundle By Name(cluster=w669, "Self Reference"=w661) -> (w668:T13)
            n268 = call <vilib>:"Add State(s) to Queue__jki_lib_state_machine.vi"("State(s) in (\"\")"=w672) -> ("States Out"=w671:string)  [unwired: 14 in]
          }
          frame "DAQ: STOP" {
            n269 = Unbundle By Name(w692) -> ("to"=w685:i32, "Self Reference"=w690:refnum<class "Lockin.DAQ.lvclass">, "state"=w688:T1)
            n270 = case shown="Default" w688 {
              selector: w688 -> [w697 w701]
              tunnel: w690 -> [w699 w709]
              tunnel: w689 -> [w696 w708]
              tunnel: [w699 w702] -> w687
              tunnel: [w698 w705] -> w686
              tunnel: w685 -> [w698 w700]
              tunnel: [w696 w704] -> w684
              tunnel: [w697 w703] -> w683
              frame "idle", "stopped" {
              }
              frame Default {
                # "stop DAQmx tasks"
                n271 = call "Lockin.DAQ.Stop.vi"("error in (no error)"=w708, "Lockin.DAQ in"=w709) -> ("error out"=w707:errorcluster, "Lockin.DAQ out"=w706:refnum<class "Lockin.DAQ.lvclass">)  [unwired: 8 in]
                n272 = case shown="No Error" w707 {
                  selector: w707 -> [w713 w716]
                  tunnel: w706 -> [w714 w717]
                  tunnel: [-1 ("to") w718] -> w705
                  tunnel: [w712 w716] -> w704
                  tunnel: [w711 w719] -> w703
                  tunnel: [w710 w717] -> w702
                  tunnel: w701 -> [_ w719]
                  tunnel: w700 -> [_ w718]
                  frame No Error {
                    w711 = State-enum."stopped" ("state")
                    n273 = call "Lockin.DAQ.getDAQState.vi"("error in (no error)"=w713, "state"=w711, "Lockin.DAQ"=w714) -> ("error out"=w712:errorcluster, "Lockin.DAQ"=w710:refnum<class "Lockin.DAQ.lvclass">)  [unwired: 7 in]
                  }
                  frame Error {
                  }
                }
              }
            }
            n274 = Bundle By Name(cluster=w692, "to"=w686, "Self Reference"=w687, "state"=w683) -> (w691:T13)
            n275 = local write "DAQ state"(w683) -> ()
            n276 = call <vilib>:"Add State(s) to Queue__jki_lib_state_machine.vi"("State(s) in (\"\")"=w695) -> ("States Out"=w694:string)  [unwired: 14 in]
          }
          frame "DAQ: CLEAR" {
            w721 = State-enum."idle" ("state")
            # "clear DAQmx tasks"
            n277 = Unbundle By Name(w729) -> ("Self Reference"=w727:refnum<class "Lockin.DAQ.lvclass">)
            n278 = call "Lockin.DAQ.Clear.vi"("error in (no error)"=w726, "Lockin.DAQ in"=w727) -> ("error out"=w725:errorcluster, "Lockin.DAQ out"=w724:refnum<class "Lockin.DAQ.lvclass">)  [unwired: 8 in]
            n279 = call "Lockin.DAQ.getDAQState.vi"("error in (no error)"=w725, "state"=w721, "Lockin.DAQ"=w724) -> ("error out"=w720:errorcluster, "Lockin.DAQ"=w722:refnum<class "Lockin.DAQ.lvclass">)  [unwired: 7 in]
            n280 = Bundle By Name(cluster=w729, "to"=-1, "Self Reference"=w722, "state"=w721) -> (w728:T13)
            n281 = local write "DAQ state"(w721) -> ()
            n282 = call <vilib>:"Add State(s) to Queue__jki_lib_state_machine.vi"("State(s) in (\"\")"=w732) -> ("States Out"=w731:string)  [unwired: 14 in]
          }
          frame "DAQ: Event" {
            # "Experimental state: generates a user event\nwhen there are a sufficient number of samples.\nUse to drive sequence instead of timeout"
            n283 = Unbundle By Name(w740) -> ("DAQmx"=w733:refnum<event-registration>)
            n284 = Unbundle By Name(w737) -> ("Self Reference"=w742:refnum<class "Lockin.DAQ.lvclass">)
            n285 = call "Lockin.DAQ.EventRegistration.vi"("error in (no error)"=w739, "DAQmx in"=w733, "Lockin.DAQ in"=w742) -> ("error out"=w738:errorcluster, "DAQmx out"=w734:refnum<event-registration>, "Lockin.DAQ out"=w735:refnum<class "Lockin.DAQ.lvclass">)  [unwired: 6 in]
            n286 = Bundle By Name(cluster=w737, "Self Reference"=w735) -> (w736:T13)
            n287 = Bundle By Name(cluster=w740, "DAQmx"=w734) -> (w741:T43)
            n288 = call <vilib>:"Add State(s) to Queue__jki_lib_state_machine.vi"("State(s) in (\"\")"=w744) -> ("States Out"=w743:string)  [unwired: 14 in]
          }
          frame "---------- DSP ----------" {
            n289 = call <vilib>:"Add State(s) to Queue__jki_lib_state_machine.vi"("State(s) in (\"\")"=w749) -> ("States Out"=w748:string)  [unwired: 14 in]
          }
          frame "DSP: Phase" {
            # "PRIVATE"
            # "PRIVATE"
            # "PRIVATE"
            n290 = Unbundle By Name(w755) -> ("Results"=w756:T12, "Self Reference"=w751:refnum<class "Lockin.DAQ.lvclass">)
            n291 = case shown="True" "reset REF" {
              tunnel: w750 -> [w767 w771]
              tunnel: w751 -> [w766 w770]
              tunnel: [w767 w769] -> w761
              tunnel: [w766 w768] -> w760
              frame False {
              }
              frame True {
                n292 = call "lockin - Set REF phase equals zero.vi"("error in (no error)"=w771, "Lockin.DAQ out"=w770) -> ("error out"=w769:errorcluster, "Lockin.DAQ"=w768:refnum<class "Lockin.DAQ.lvclass">)  [unwired: 8 in]
              }
            }
            n293 = case shown="True" "autophase?\n(experimental)" {
              tunnel: w756 -> [_ w774]
              tunnel: w761 -> [w773 w778]
              tunnel: w760 -> [w772 w777]
              tunnel: [w773 w776] -> w759
              tunnel: [w772 w775] -> w757
              frame False {
              }
              frame True {
                n294 = call "4461 Autophase.vi"("error in (no error)"=w778, "Results"=w774, "Lockin.DAQ in"=w777) -> ("error out"=w776:errorcluster, "Lockin.DAQ out"=w775:refnum<class "Lockin.DAQ.lvclass">)  [unwired: 7 in]
              }
            }
            n295 = call "4461 Replace AO Ch.vi"("error in (no error)"=w759, "Lockin.DAQ (NEW)"=w757, "Lockin.DAQ (OLD)"=w751) -> ("error out"=w753:errorcluster, "Lockin.DAQ out"=w752:refnum<class "Lockin.DAQ.lvclass">)  [unwired: 7 in]
            n296 = Bundle By Name(cluster=w755, "Self Reference"=w752) -> (w754:T13)
            n297 = call <vilib>:"Add State(s) to Queue__jki_lib_state_machine.vi"("State(s) in (\"\")"=w765) -> ("States Out"=w764:string)  [unwired: 14 in]
          }
          frame "DSP: Filter" {
            # "publish waveforms"
            n298 = Unbundle By Name(w824) -> ("Self Reference"=w780:refnum<class "Lockin.DAQ.lvclass">, "AO"=w792:waveform(dbl)[], "Reference"=w787:T38, "AI"=w801:waveform(dbl)[], "DAQ Offset"=w793:dbl[])
            n299 = Unbundle(w787) -> ("X"=w786:waveform(dbl)[], "Y"=w785:waveform(dbl)[])
            n300 = call "decimate_waveforms.vi"("error in (no error)"=w802, "WFM"=w792, "LockinDAQ"=w780) -> ("error out"=w804:errorcluster, "WFM out"=w803:waveform(dbl)[], "LockinDAQ out"=w797:refnum<class "Lockin.DAQ.lvclass">)  [unwired: 6 in]
            n301 = call "decimate_waveforms.vi"("error in (no error)"=w802, "WFM"=w801, "LockinDAQ"=w780) -> ("error out"=w800:errorcluster, "WFM out"=w806:waveform(dbl)[], "LockinDAQ out"=w807:refnum<class "Lockin.DAQ.lvclass">)  [unwired: 6 in]
            n302 = call "decimate_waveforms.vi"("error in (no error)"=w802, "WFM"=w785, "LockinDAQ"=w780) -> ("error out"=w794:errorcluster, "WFM out"=w798:waveform(dbl)[], "LockinDAQ out"=w796:refnum<class "Lockin.DAQ.lvclass">)  [unwired: 6 in]
            n303 = call "decimate_waveforms.vi"("WFM"=w786, "LockinDAQ"=w780) -> ("error out"=w791:errorcluster, "WFM out"=w790:waveform(dbl)[])  [unwired: 7 in, 1 out]
            n304 = call "Subtract DAQ Offset.vi"("error in (no error)"=w800, "DAQ Offset"=w793, "WFM in"=w806, "Lockin.DAQ"=w807) -> ("error out"=w799:errorcluster, "WFM out"=w805:waveform(dbl)[], "Lockin.DAQ out"=w795:refnum<class "Lockin.DAQ.lvclass">)  [unwired: 5 in]
            n305 = case shown="True" "LP filter?" {
              tunnel: w805 -> [w835 w855]
              tunnel: [w835 w851] -> w812
              tunnel: w799 -> [w834 w853]
              tunnel: [w834 w852] -> w811
              tunnel: "LP Cutoff (Hz)" -> [_ w854]
              tunnel: "LP Cutoff (Hz)" -> [_ w850]
              tunnel: "LP Cutoff (Hz)" -> [_ w849]
              tunnel: w803 -> [w833 w848]
              tunnel: [w833 w847] -> w816
              tunnel: w798 -> [w831 w846]
              tunnel: [w831 w845] -> w814
              tunnel: w804 -> [w832 w844]
              tunnel: [w832 w843] -> w815
              tunnel: [w830 w842] -> w813
              tunnel: w794 -> [w830 w841]
              tunnel: "LP Cutoff (Hz)" -> [_ w836]
              tunnel: w790 -> [w828 w837]
              tunnel: [w828 w838] -> w788
              tunnel: [w829 w839] -> w789
              tunnel: w791 -> [w829 w840]
              frame False {
              }
              frame True {
                n306 = call "Prefilter_LP.vi"("error in (no error)"=w844, "high cutoff freq [Hz]"=w849, "WFM in"=w848) -> ("error out"=w843:errorcluster, "WFM out"=w847:waveform(dbl)[])  [unwired: 7 in]
                n307 = call "Prefilter_LP.vi"("error in (no error)"=w841, "high cutoff freq [Hz]"=w850, "WFM in"=w846) -> ("error out"=w842:errorcluster, "WFM out"=w845:waveform(dbl)[])  [unwired: 7 in]
                n308 = call "Prefilter_LP.vi"("error in (no error)"=w853, "high cutoff freq [Hz]"=w854, "WFM in"=w855) -> ("error out"=w852:errorcluster, "WFM out"=w851:waveform(dbl)[])  [unwired: 7 in]
                n309 = call "Prefilter_LP.vi"("error in (no error)"=w840, "high cutoff freq [Hz]"=w836, "WFM in"=w837) -> ("error out"=w839:errorcluster, "WFM out"=w838:waveform(dbl)[])  [unwired: 7 in]
              }
            }
            n310 = case shown="False" "60 Hz Prefilter?" {
              tunnel: w812 -> [w863 w879]
              tunnel: [w863 w878] -> w808
              tunnel: w811 -> [w862 w877]
              tunnel: [w862 w876] -> w810
              tunnel: w816 -> [w858 w875]
              tunnel: [w858 w874] -> w809
              tunnel: w814 -> [w860 w873]
              tunnel: [w860 w872] -> w783
              tunnel: w813 -> [w861 w871]
              tunnel: w815 -> [w859 w870]
              tunnel: [w859 w869] -> _
              tunnel: [w861 w868] -> w782
              tunnel: w788 -> [w856 w864]
              tunnel: [w856 w865] -> w784
              tunnel: w789 -> [w857 w866]
              tunnel: [w857 w867] -> _
              frame False {
              }
              frame True {
                n311 = call "Prefilter_60Hz_Notch.vi"("error in (no error)"=w870, "Array in"=w875) -> ("error out"=w869:errorcluster, "Array out"=w874:waveform(dbl)[])  [unwired: 8 in]
                n312 = call "Prefilter_60Hz_Notch.vi"("error in (no error)"=w871, "Array in"=w873) -> ("error out"=w868:errorcluster, "Array out"=w872:waveform(dbl)[])  [unwired: 8 in]
                n313 = call "Prefilter_60Hz_Notch.vi"("error in (no error)"=w877, "Array in"=w879) -> ("error out"=w876:errorcluster, "Array out"=w878:waveform(dbl)[])  [unwired: 8 in]
                n314 = call "Prefilter_60Hz_Notch.vi"("error in (no error)"=w866, "Array in"=w864) -> ("error out"=w867:errorcluster, "Array out"=w865:waveform(dbl)[])  [unwired: 8 in]
              }
            }
            n315 = Bundle("Array out"=w784, "Array out"=w783) -> (w779:T46)  [unwired: 1 in]
            n316 = call "Lockin.DAQ.getAO.vi"("get AO"=w809, "Lockin.DAQ"=w797) -> ("error out"=w820:errorcluster)  [unwired: 8 in, 1 out]
            n317 = call "Lockin.DAQ.getAI.vi"("error in (no error)"=w810, "getAI"=w808, "Lockin.DAQ"=w795) -> ("error out"=w819:errorcluster)  [unwired: 7 in, 1 out]
            n318 = call "Lockin.DAQ.getREF.vi"("error in (no error)"=w782, "getREF"=w779, "Lockin.DAQ"=w796) -> ("error out"=w821:errorcluster)  [unwired: 7 in, 1 out]
            n319 = Bundle By Name(cluster=w824, "AO"=w809, "Reference"=w779, "AI"=w808) -> (w823:T13)
            n320 = Merge Errors(w820, w821, w819) -> (w818:errorcluster)
            n321 = call <vilib>:"Add State(s) to Queue__jki_lib_state_machine.vi"("State(s) in (\"\")"=w827) -> ("States Out"=w826:string)  [unwired: 14 in]
          }
          frame "DSP: Lockin" {
            # "publish Results"
            # "lockin demodulation"
            n322 = Unbundle By Name(w896) -> ("Self Reference"=w883:refnum<class "Lockin.DAQ.lvclass">, "AI"=w882:waveform(dbl)[], "Reference"=w880:T38)
            n323 = call <userlib>:"Tick Count (ms)__ogtk.vi"("error in (no error)"=w894) -> ("error out"=w881:errorcluster, "millisecond timer value"=w887:u32)  [unwired: 9 in]
            n324 = call "Lockin Engine.vi"("error in (no error)"=w881, "Reference"=w880, "AI Waveforms"=w882, "Lockin.DAQ"=w883) -> ("error out"=w891:errorcluster, "SweepResults"=w885:T6, "Averaged Results (X,Y,R,Theta,Mean)"=w884:T12, "Lockin.DAQ"=w893:refnum<class "Lockin.DAQ.lvclass">)  [unwired: 4 in]
            n325 = call "Lockin.DAQ.getResults.vi"("error in (no error)"=w891, "Results"=w884, "Lockin.DAQ"=w893) -> ("error out"=w890:errorcluster, "Lockin.DAQ out"=w892:refnum<class "Lockin.DAQ.lvclass">)  [unwired: 7 in]
            n326 = Bundle By Name(cluster=w896, "Self Reference"=w892, "Results"=w884, "SweepResults [i]"=w885) -> (w895:T13)
            n327 = call <userlib>:"Tick Count (ms)__ogtk.vi"("error in (no error)"=w890) -> ("error out"=w889:errorcluster, "millisecond timer value"=w888:u32)  [unwired: 9 in]
            n328 = Subtract(x=w888, y=w887) -> (x-y=→"Lockin (ms)":u32)
            n329 = call <vilib>:"Add State(s) to Queue__jki_lib_state_machine.vi"("State(s) in (\"\")"=w899) -> ("States Out"=w898:string)  [unwired: 14 in]
          }
          frame "DSP: Measure DAQ Offset" {
            w901 = FALSE ("measureOffset")
            # "remove any existing offset\nbefore calculating new offset"
            # "reset indicator after measuring"
            n330 = Unbundle By Name(w912) -> ("Self Reference"=w902:refnum<class "Lockin.DAQ.lvclass">, "AI"=w903:waveform(dbl)[], "DAQ Offset"=w908:dbl[])
            n331 = Negate(x=w908) -> (-x=w907:dbl[])
            n332 = call "Subtract DAQ Offset.vi"("error in (no error)"=w905, "DAQ Offset"=w907, "WFM in"=w903, "Lockin.DAQ"=w902) -> ("error out"=w904:errorcluster, "WFM out"=w906:waveform(dbl)[])  [unwired: 5 in, 1 out]
            n333 = call-poly <vilib>:"Basic Averaged DC-RMS.vi"("reset"=TRUE, "error in (no error)"=w904, "signals in"=w906) -> ("error out"=w909:errorcluster, "DC values"=w910:dbl[])  [unwired: 5 in, 2 out]
            n334 = Bundle By Name(cluster=w912, "DAQ Offset"=w910, "Measure Offset"=w901) -> (w911:T13)
            n335 = local write "measure offset"(w901) -> ()
            n336 = call <vilib>:"Add State(s) to Queue__jki_lib_state_machine.vi"("State(s) in (\"\")"=w915) -> ("States Out"=w914:string)  [unwired: 14 in]
          }
          frame "DSP: Zero DAQ Offset" {
            # "reset indicator after zeroing"
            n337 = Unbundle By Name(w918) -> ("AI"=w917:waveform(dbl)[])
            n338 = for {
              tunnel: w917 -> [_] mode=indexing
              tunnel: [0.0] -> w916 mode=indexing
            }
            n339 = Bundle By Name(cluster=w918, "DAQ Offset"=w916) -> (w920:T13)
            n340 = local write "zero offset"(FALSE ("measureOffset")) -> ()
            n341 = call <vilib>:"Add State(s) to Queue__jki_lib_state_machine.vi"("State(s) in (\"\")"=w924) -> ("States Out"=w923:string)  [unwired: 14 in]
          }
          frame "---------- Sweep ----------" {
            n342 = call <vilib>:"Add State(s) to Queue__jki_lib_state_machine.vi"("State(s) in (\"\")"=w930) -> ("States Out"=w929:string)  [unwired: 14 in]
          }
          frame "Sweep: Initialize" {
            w932 = waveform(dbl)[] [] ("Sweep_AO")
            w937 = State-enum."sweeping" ("state")
            n343 = Unbundle By Name(w940) -> ("Self Reference"=w933:refnum<class "Lockin.DAQ.lvclass">)
            n344 = call "Lockin.DAQ.getDAQState.vi"("error in (no error)"=w935, "state"=w937, "Lockin.DAQ"=w933) -> ("error out"=w938:errorcluster, "Lockin.DAQ"=w934:refnum<class "Lockin.DAQ.lvclass">)  [unwired: 7 in]
            n345 = Bundle By Name(cluster=w940, "Self Reference"=w934, "SweepResults []"=T6 {"X results"=[], "Y Results"=[]} ("All Results []"), "Sweep_AO"=w932, "Sweep_AI"=w932, "state"=w937, "sweep index"=0) -> (w939:T13)
            n346 = call <vilib>:"Add State(s) to Queue__jki_lib_state_machine.vi"("State(s) in (\"\")"=w943) -> ("States Out"=w942:string)  [unwired: 14 in]
          }
          frame "Sweep: Set Initial" {
            # "1: Set Initial Vstart"
            n347 = flat-sequence {
              tunnel: [w952] -> w947
              tunnel: w945 -> [w951]
              tunnel: [w951] -> w946
              frame #0 {
                n348 = Get Date/Time In Seconds() -> (seconds since 1Jan1904=w952:timestamp)
              }
            }
            n349 = call <vilib>:"Add State(s) to Queue__jki_lib_state_machine.vi"("State(s) in (\"\")"=w950) -> ("States Out"=w949:string)  [unwired: 14 in]
            "Sweep Start" <- w947
          }
          frame "Sweep: Wait" {
            n350 = Unbundle By Name(w960) -> ("sweep index"=w965:i32, "Self Reference"=w957:refnum<class "Lockin.DAQ.lvclass">)
            n351 = local read "Sweep Start"() -> (w954:timestamp)
            n352 = Equal To 0?(x=w965) -> (x = 0?=w964:bool)
            n353 = Get Date/Time In Seconds() -> (seconds since 1Jan1904=w955:timestamp)
            "Sweep Wait Time" <- w955
            n354 = Unbundle By Name(w957) -> ("Initial Wait (s)"=w966:dbl)
            n355 = Subtract(x=w955, y=w954) -> (x-y=→"waiting (s)":dbl)
            n356 = Multiply(x=w966, y=1000.0) -> (x*y=w962:dbl)
            n357 = call <userlib>:"Periodic Trigger__ogtk.vi"("time (ms)"=w962, "reset"=w964) -> ("Triggered"=w963:bool)  [unwired: 11 in, 2 out]
            n358 = case shown="False" w963 {
              tunnel: [1 ("sweep index") 2 ("sweep index")] -> w961
              frame False {
              }
              frame True {
              }
            }
            n359 = Bundle By Name(cluster=w960, "sweep index"=w961) -> (w959:T13)
            n360 = call <vilib>:"Add State(s) to Queue__jki_lib_state_machine.vi"("State(s) in (\"\")"=w969) -> ("States Out"=w968:string)  [unwired: 14 in]
          }
          frame "Sweep: Configure Sweep" {
            # "2. Setup Sweep from Vstart to Vend in Time_sweep"
            n361 = Bundle By Name(cluster=w975, "sweep index"=3) -> (w974:T13)
            n362 = call <vilib>:"Add State(s) to Queue__jki_lib_state_machine.vi"("State(s) in (\"\")"=w978) -> ("States Out"=w977:string)  [unwired: 14 in]
          }
          frame "Sweep: Done Sweeping?" {
            # "add some overhead time"
            # "#todo\ndo something more sophisticated...like compare 1st and last points of array\nand decide if next write will be more"
            n363 = Unbundle By Name(w997) -> ("Self Reference"=w981:refnum<class "Lockin.DAQ.lvclass">)
            n364 = Unbundle By Name(w981) -> ("AO Channels"=w980:T20, "Sweep Time (s)"=w994:dbl, "Initial Wait (s)"=w982:dbl)
            n365 = flat-sequence {
              tunnel: [w1004] -> w987
              tunnel: [w1003] -> w991
              tunnel: w990 -> [w1003]
              frame #0 {
                n366 = Get Date/Time In Seconds() -> (seconds since 1Jan1904=w1004:timestamp)
              }
            }
            n367 = local read "Sweep Wait Time"() -> (w986:timestamp)
            n368 = for {
              tunnel: w980 -> [w1002] mode=indexing
              tunnel: [w1001] -> w979 mode=indexing
              n369 = Unbundle By Name(w1002) -> ("Sweeping?"=w1001:bool)
            }
            n370 = Subtract(x=w987, y=w986) -> (x-y=w985:dbl)
            "sweeping" <- w985
            n371 = Add(x=w994, y=w982) -> (x+y=w984:dbl)
            n372 = Add(x=w984, y=10.0) -> (x+y=w993:dbl)
            n373 = Not(x=w979) -> (.not. x?=w988:bool[])
            n374 = And Array Elements(Boolean array=w988) -> (logical AND=w995:bool)
            "done sweep?" <- w995
            n375 = Greater?(x=w985, y=w993) -> (0:w992:bool)
            "timeout?" <- w992
            n376 = Or(x=w995, y=w992) -> (x .or. y?=w989:bool)
            n377 = case shown="True" w989 {
              tunnel: w997 -> [w1005 w1008]
              tunnel: [w1005 w1007] -> w996
              frame False {
              }
              frame True {
                n378 = Bundle By Name(cluster=w1008, "sweep index"=4) -> (w1007:T13)
              }
            }
            n379 = call <vilib>:"Add State(s) to Queue__jki_lib_state_machine.vi"("State(s) in (\"\")"=w1000) -> ("States Out"=w999:string)  [unwired: 14 in]
            "Sweeping Time" <- w987
          }
          frame "Sweep: Save" {
            # "#todo\nthis one needs to be more dynamic\nin case we are sweeping f or phase"
            # "Gather most recent results array and add to previous results"
            n380 = Unbundle By Name(w1022) -> ("sweep index"=w1009:i32, "SweepResults [i].X results"=w1025:waveform(dbl)[], "SweepResults [i].X results"=w1024:waveform(dbl)[], "SweepResults [i].Y Results"=w1011:waveform(dbl)[], "SweepResults [i].Y Results"=w1010:waveform(dbl)[], "Sweep_AO"=w1020:waveform(dbl)[], "AO"=w1018:waveform(dbl)[], "Sweep_AI"=w1019:waveform(dbl)[], "AI"=w1013:waveform(dbl)[])
            n381 = case shown="Default" w1009 {
              tunnel: w1025 -> [w1029 w1043]
              tunnel: w1024 -> [_ w1041]
              tunnel: [w1029 w1042] -> w1023
              tunnel: w1020 -> [w1033 w1050]
              tunnel: w1019 -> [w1032 w1049]
              tunnel: w1018 -> [_ w1048]
              tunnel: [w1033 w1034] -> w1017
              tunnel: [w1032 w1047] -> w1016
              tunnel: [w1031 w1046] -> w1015
              tunnel: w1014 -> [w1031 w1036]
              tunnel: w1013 -> [_ w1045]
              tunnel: [w1030 w1040] -> w1012
              tunnel: w1011 -> [w1030 w1039]
              tunnel: w1010 -> [_ w1038]
              frame 4 {
              }
              frame Default {
                n382 = call "Append Multiple Waveforms.vi"("error in (no error)"=w1036, "Waveform B []"=w1041, "Waveforrm A []"=w1043) -> ("error out"=w1035:errorcluster, "Waveform out []"=w1042:waveform(dbl)[])  [unwired: 7 in]
                n383 = call "Append Multiple Waveforms.vi"("error in (no error)"=w1035, "Waveform B []"=w1038, "Waveforrm A []"=w1039) -> ("error out"=w1037:errorcluster, "Waveform out []"=w1040:waveform(dbl)[])  [unwired: 7 in]
                n384 = call "Append Multiple Waveforms.vi"("error in (no error)"=w1037, "Waveform B []"=w1048, "Waveforrm A []"=w1050) -> ("error out"=w1044:errorcluster, "Waveform out []"=w1034:waveform(dbl)[])  [unwired: 7 in]
                n385 = call "Append Multiple Waveforms.vi"("error in (no error)"=w1044, "Waveform B []"=w1045, "Waveforrm A []"=w1049) -> ("error out"=w1046:errorcluster, "Waveform out []"=w1047:waveform(dbl)[])  [unwired: 7 in]
              }
            }
            n386 = Bundle By Name(cluster=w1022, "SweepResults [i].X results"=w1023, "SweepResults [i].Y Results"=w1012, "Sweep_AO"=w1017, "Sweep_AI"=w1016) -> (w1021:T13)
            n387 = call <vilib>:"Add State(s) to Queue__jki_lib_state_machine.vi"("State(s) in (\"\")"=w1028) -> ("States Out"=w1027:string)  [unwired: 14 in]
          }
          frame "Sweep: Stop" {
            w1055 = State-enum."started" ("state")
            n388 = Unbundle By Name(w1065) -> ("Self Reference"=w1061:refnum<class "Lockin.DAQ.lvclass">, "SweepResults []"=w1052:T6, "Sweep_AO"=w1053:waveform(dbl)[], "Sweep_AI"=w1054:waveform(dbl)[])
            n389 = call "Lockin.DAQ.getSweepResults.vi"("error in (no error)"=w1063, "getSweepResults"=w1052, "LockinDAQ"=w1061) -> ("error out"=w1057:errorcluster, "LockinDAQ"=w1059:refnum<class "Lockin.DAQ.lvclass">)  [unwired: 7 in]
            n390 = Bundle("Sweep_AO"=w1053, "Sweep_AI"=w1054) -> (w1051:T47)  [unwired: 1 in]
            n391 = call "Lockin.DAQ.getIVSweepResults.vi"("error in (no error)"=w1057, "SweepWFMs"=w1051, "LockinDAQ"=w1059) -> ("error out"=w1056:errorcluster, "LockinDAQ out"=w1058:refnum<class "Lockin.DAQ.lvclass">)  [unwired: 7 in]
            n392 = call "Lockin.DAQ.getDAQState.vi"("error in (no error)"=w1056, "state"=w1055, "Lockin.DAQ"=w1058) -> ("error out"=w1064:errorcluster, "Lockin.DAQ"=w1062:refnum<class "Lockin.DAQ.lvclass">)  [unwired: 7 in]
            n393 = Bundle By Name(cluster=w1065, "Self Reference"=w1062, "state"=w1055, "sweep index"=-1) -> (w1066:T13)
            n394 = call <vilib>:"Add State(s) to Queue__jki_lib_state_machine.vi"("State(s) in (\"\")"=w1069) -> ("States Out"=w1068:string)  [unwired: 14 in]
          }
          frame "---------- Generate ----------" {
            n395 = call <vilib>:"Add State(s) to Queue__jki_lib_state_machine.vi"("State(s) in (\"\")"=w1074) -> ("States Out"=w1073:string)  [unwired: 14 in]
          }
          frame "Generate: Generate" {
            w1078 = FALSE ("Reset Phase")
            n396 = Unbundle By Name(w1094) -> ("Self Reference"=w1084:refnum<class "Lockin.DAQ.lvclass">, "Measure Offset"=w1075:bool, "Reset Phase"=w1076:bool, "sweep index"=w1077:i32)
            n397 = call <userlib>:"Tick Count (ms)__ogtk.vi"("error in (no error)"=w1091) -> ("error out"=w1089:errorcluster, "millisecond timer value"=w1086:u32)  [unwired: 9 in]
            n398 = call "lockin - zero amplitude.vi"("measure\noffset?"=w1075, "error in (no error)"=w1089, "Lockin.DAQ"=w1084) -> ("error out"=w1090:errorcluster, "Lockin.DAQ out"=w1083:refnum<class "Lockin.DAQ.lvclass">)  [unwired: 7 in]
            n399 = call "Lockin.DAQ.Generate.Waveforms.vi"("sweep index"=w1077, "Reset Phase?"=w1076, "error in (no error)"=w1090, "Lockin.DAQ"=w1083) -> ("error out"=w1081:errorcluster, "Reference"=w1079:T38, "AO []"=w1092:waveform(dbl)[], "Lockin.DAQ"=w1080:refnum<class "Lockin.DAQ.lvclass">)  [unwired: 4 in]
            n400 = call <userlib>:"Tick Count (ms)__ogtk.vi"("error in (no error)"=w1081) -> ("error out"=w1088:errorcluster, "millisecond timer value"=w1087:u32)  [unwired: 9 in]
            n401 = Subtract(x=w1087, y=w1086) -> (x-y=→"WFM Generation (ms)":u32)
            n402 = Bundle By Name(cluster=w1094, "Self Reference"=w1080, "AO"=w1092, "Reference"=w1079, "Reset Phase"=w1078) -> (w1093:T13)
            n403 = local write "Reset Phase?"(w1078) -> ()
            n404 = call <vilib>:"Add State(s) to Queue__jki_lib_state_machine.vi"("State(s) in (\"\")"=w1082) -> ("States Out"=w1096:string)  [unwired: 14 in]
          }
        }
      }
    }
    frame Error {
    }
  }
  n405 = call-parent "Process.vi"("error in"=w7, "SMO"=w6) -> ("error out"=w4:errorcluster, "SMO out"=→"LockinDAQ out":refnum<class "Lockin.DAQ.lvclass">)  [unwired: 8 in]
  n406 = Merge Errors(w4, w3) -> (→"error out":errorcluster)
